vi "19_2.vi"() -> ()   [LabVIEW 2018]
uses:
  <userlib>/_OpenG.lib/array/array.llb/Remove Duplicates from 1D Array (String)__ogtk.vi
  <vilib>/regexp/Match Regular Expression.xnode
panel:
  out "size(s)":i32=311
  out "Array":i16[](array[numeric])=[190, 18, 8, 3, 0, 0, 0, 0, 0, 0, 37, 9, 0, 0, 0, 0, 0, 0, 0, 0, 23, 7, 0, 0, 0, 0, 0, 0, 0, 0, 10, 1, 0, 0, 0, 0, 0, 0, 0, 0, 5, 0, 0, 0, 0, 0, 0, 0, 0, 0, 0, 0, 0, 0, 0, 0, 0, 0, 0, 0, 0, 0, 0, 0, 0, 0, 0, 0, 0, 0, 0, 0, 0, 0, 0, 0, 0, 0, 0, 0, 0, 0, 0, 0, 0, 0, 0, 0, 0, 0, 0, 0, 0, 0, 0, 0, 0, 0, 0, 0]
  out "sum":i16
  out "String":string="((((a((a(b(aa|ba)|a(ab|aa))|b(b(bb|aa)|a(ba)))a|(((ab|ba)b)b|((aa|ba)b|((a|b)(a|b))a)a)b)|b((a(a(ba|a(a|b))|b((a|b)(a|b)))|b((ba)b|(bb|aa)a))a|((b(bb)|a(ab|ba))b|(b(bb|aa)|a(ba))a)b))a|(b(b(a(b(bb|aa)|a(ab|ba))|b(b(bb|aa)|a(ba)))|a(((bb)a|(bb|aa)b)a|((bb|aa)a|(aa|ba)b)b))|a(a(b(a(bb|aa)|b(aa|ba))|a((bb|ab)a|((a|b)b|ba)b))|b((a(aa|ba))a|((b(a|b)|aa)b|(ba)a)b)))b)a|(a(a(a((b(ba)|a(bb|aa))b|(b(bb|ab)|a(aa))a)|b(((bb|ab)b|(b(a|b)|aa)a)b|(b(bb|aa)|a(ab|ba))a))|b((a((b(a|b)|aa)b|(ba)a)|b((ba|bb)b|(ba|a(a|b))a))a|(b(b(ba)|a(bb|ab))|a((ba)b|(bb|aa)a))b))|b(a((((ba|bb)b|(ab|aa)a)a|((ba|a(a|b))(a|b))b)b|(((aa|ba)a|(ba|a(a|b))b)b|(a(aa|ba)|b(aa))a)a)|b((a(b((a|b)(a|b))|a(aa|ba))|b((ab|ba)b|(bb|ab)a))a|(a((ba|bb)a|(b(a|b)|aa)b)|b(((a|b)(a|b))b|(ba)a))b)))b)(((a((a(b(aa|ba)|a(ab|aa))|b(b(bb|aa)|a(ba)))a|(((ab|ba)b)b|((aa|ba)b|((a|b)(a|b))a)a)b)|b((a(a(ba|a(a|b))|b((a|b)(a|b)))|b((ba)b|(bb|aa)a))a|((b(bb)|a(ab|ba))b|(b(bb|aa)|a(ba))a)b))a|(b(b(a(b(bb|aa)|a(ab|ba))|b(b(bb|aa)|a(ba)))|a(((bb)a|(bb|aa)b)a|((bb|aa)a|(aa|ba)b)b))|a(a(b(a(bb|aa)|b(aa|ba))|a((bb|ab)a|((a|b)b|ba)b))|b((a(aa|ba))a|((b(a|b)|aa)b|(ba)a)b)))b)a|(a(a(a((b(ba)|a(bb|aa))b|(b(bb|ab)|a(aa))a)|b(((bb|ab)b|(b(a|b)|aa)a)b|(b(bb|aa)|a(ab|ba))a))|b((a((b(a|b)|aa)b|(ba)a)|b((ba|bb)b|(ba|a(a|b))a))a|(b(b(ba)|a(bb|ab))|a((ba)b|(bb|aa)a))b))|b(a((((ba|bb)b|(ab|aa)a)a|((ba|a(a|b))(a|b))b)b|(((aa|ba)a|(ba|a(a|b))b)b|(a(aa|ba)|b(aa))a)a)|b((a(b((a|b)(a|b))|a(aa|ba))|b((ab|ba)b|(bb|ab)a))a|(a((ba|bb)a|(b(a|b)|aa)b)|b(((a|b)(a|b))b|(ba)a))b)))b)(((a((a(b(aa|ba)|a(ab|aa))|b(b(bb|aa)|a(ba)))a|(((ab|ba)b)b|((aa|ba)b|((a|b)(a|b))a)a)b)|b((a(a(ba|a(a|b))|b((a|b)(a|b)))|b((ba)b|(bb|aa)a))a|((b(bb)|a(ab|ba))b|(b(bb|aa)|a(ba))a)b))a|(b(b(a(b(bb|aa)|a(ab|ba))|b(b(bb|aa)|a(ba)))|a(((bb)a|(bb|aa)b)a|((bb|aa)a|(aa|ba)b)b))|a(a(b(a(bb|aa)|b(aa|ba))|a((bb|ab)a|((a|b)b|ba)b))|b((a(aa|ba))a|((b(a|b)|aa)b|(ba)a)b)))b)a|(a(a(a((b(ba)|a(bb|aa))b|(b(bb|ab)|a(aa))a)|b(((bb|ab)b|(b(a|b)|aa)a)b|(b(bb|aa)|a(ab|ba))a))|b((a((b(a|b)|aa)b|(ba)a)|b((ba|bb)b|(ba|a(a|b))a))a|(b(b(ba)|a(bb|ab))|a((ba)b|(bb|aa)a))b))|b(a((((ba|bb)b|(ab|aa)a)a|((ba|a(a|b))(a|b))b)b|(((aa|ba)a|(ba|a(a|b))b)b|(a(aa|ba)|b(aa))a)a)|b((a(b((a|b)(a|b))|a(aa|ba))|b((ab|ba)b|(bb|ab)a))a|(a((ba|bb)a|(b(a|b)|aa)b)|b(((a|b)(a|b))b|(ba)a))b)))b)(((a((a(b(aa|ba)|a(ab|aa))|b(b(bb|aa)|a(ba)))a|(((ab|ba)b)b|((aa|ba)b|((a|b)(a|b))a)a)b)|b((a(a(ba|a(a|b))|b((a|b)(a|b)))|b((ba)b|(bb|aa)a))a|((b(bb)|a(ab|ba))b|(b(bb|aa)|a(ba))a)b))a|(b(b(a(b(bb|aa)|a(ab|ba))|b(b(bb|aa)|a(ba)))|a(((bb)a|(bb|aa)b)a|((bb|aa)a|(aa|ba)b)b))|a(a(b(a(bb|aa)|b(aa|ba))|a((bb|ab)a|((a|b)b|ba)b))|b((a(aa|ba))a|((b(a|b)|aa)b|(ba)a)b)))b)a|(a(a(a((b(ba)|a(bb|aa))b|(b(bb|ab)|a(aa))a)|b(((bb|ab)b|(b(a|b)|aa)a)b|(b(bb|aa)|a(ab|ba))a))|b((a((b(a|b)|aa)b|(ba)a)|b((ba|bb)b|(ba|a(a|b))a))a|(b(b(ba)|a(bb|ab))|a((ba)b|(bb|aa)a))b))|b(a((((ba|bb)b|(ab|aa)a)a|((ba|a(a|b))(a|b))b)b|(((aa|ba)a|(ba|a(a|b))b)b|(a(aa|ba)|b(aa))a)a)|b((a(b((a|b)(a|b))|a(aa|ba))|b((ab|ba)b|(bb|ab)a))a|(a((ba|bb)a|(b(a|b)|aa)b)|b(((a|b)(a|b))b|(ba)a))b)))b)(((a((a(b(aa|ba)|a(ab|aa))|b(b(bb|aa)|a(ba)))a|(((ab|ba)b)b|((aa|ba)b|((a|b)(a|b))a)a)b)|b((a(a(ba|a(a|b))|b((a|b)(a|b)))|b((ba)b|(bb|aa)a))a|((b(bb)|a(ab|ba))b|(b(bb|aa)|a(ba))a)b))a|(b(b(a(b(bb|aa)|a(ab|ba))|b(b(bb|aa)|a(ba)))|a(((bb)a|(bb|aa)b)a|((bb|aa)a|(aa|ba)b)b))|a(a(b(a(bb|aa)|b(aa|ba))|a((bb|ab)a|((a|b)b|ba)b))|b((a(aa|ba))a|((b(a|b)|aa)b|(ba)a)b)))b)a|(a(a(a((b(ba)|a(bb|aa))b|(b(bb|ab)|a(aa))a)|b(((bb|ab)b|(b(a|b)|aa)a)b|(b(bb|aa)|a(ab|ba))a))|b((a((b(a|b)|aa)b|(ba)a)|b((ba|bb)b|(ba|a(a|b))a))a|(b(b(ba)|a(bb|ab))|a((ba)b|(bb|aa)a))b))|b(a((((ba|bb)b|(ab|aa)a)a|((ba|a(a|b))(a|b))b)b|(((aa|ba)a|(ba|a(a|b))b)b|(a(aa|ba)|b(aa))a)a)|b((a(b((a|b)(a|b))|a(aa|ba))|b((ab|ba)b|(bb|ab)a))a|(a((ba|bb)a|(b(a|b)|aa)b)|b(((a|b)(a|b))b|(ba)a))b)))b)(((a((a(b(aa|ba)|a(ab|aa))|b(b(bb|aa)|a(ba)))a|(((ab|ba)b)b|((aa|ba)b|((a|b)(a|b))a)a)b)|b((a(a(ba|a(a|b))|b((a|b)(a|b)))|b((ba)b|(bb|aa)a))a|((b(bb)|a(ab|ba))b|(b(bb|aa)|a(ba))a)b))a|(b(b(a(b(bb|aa)|a(ab|ba))|b(b(bb|aa)|a(ba)))|a(((bb)a|(bb|aa)b)a|((bb|aa)a|(aa|ba)b)b))|a(a(b(a(bb|aa)|b(aa|ba))|a((bb|ab)a|((a|b)b|ba)b))|b((a(aa|ba))a|((b(a|b)|aa)b|(ba)a)b)))b)a|(a(a(a((b(ba)|a(bb|aa))b|(b(bb|ab)|a(aa))a)|b(((bb|ab)b|(b(a|b)|aa)a)b|(b(bb|aa)|a(ab|ba))a))|b((a((b(a|b)|aa)b|(ba)a)|b((ba|bb)b|(ba|a(a|b))a))a|(b(b(ba)|a(bb|ab))|a((ba)b|(bb|aa)a))b))|b(a((((ba|bb)b|(ab|aa)a)a|((ba|a(a|b))(a|b))b)b|(((aa|ba)a|(ba|a(a|b))b)b|(a(aa|ba)|b(aa))a)a)|b((a(b((a|b)(a|b))|a(aa|ba))|b((ab|ba)b|(bb|ab)a))a|(a((ba|bb)a|(b(a|b)|aa)b)|b(((a|b)(a|b))b|(ba)a))b)))b)(((a((a(b(aa|ba)|a(ab|aa))|b(b(bb|aa)|a(ba)))a|(((ab|ba)b)b|((aa|ba)b|((a|b)(a|b))a)a)b)|b((a(a(ba|a(a|b))|b((a|b)(a|b)))|b((ba)b|(bb|aa)a))a|((b(bb)|a(ab|ba))b|(b(bb|aa)|a(ba))a)b))a|(b(b(a(b(bb|aa)|a(ab|ba))|b(b(bb|aa)|a(ba)))|a(((bb)a|(bb|aa)b)a|((bb|aa)a|(aa|ba)b)b))|a(a(b(a(bb|aa)|b(aa|ba))|a((bb|ab)a|((a|b)b|ba)b))|b((a(aa|ba))a|((b(a|b)|aa)b|(ba)a)b)))b)a|(a(a(a((b(ba)|a(bb|aa))b|(b(bb|ab)|a(aa))a)|b(((bb|ab)b|(b(a|b)|aa)a)b|(b(bb|aa)|a(ab|ba))a))|b((a((b(a|b)|aa)b|(ba)a)|b((ba|bb)b|(ba|a(a|b))a))a|(b(b(ba)|a(bb|ab))|a((ba)b|(bb|aa)a))b))|b(a((((ba|bb)b|(ab|aa)a)a|((ba|a(a|b))(a|b))b)b|(((aa|ba)a|(ba|a(a|b))b)b|(a(aa|ba)|b(aa))a)a)|b((a(b((a|b)(a|b))|a(aa|ba))|b((ab|ba)b|(bb|ab)a))a|(a((ba|bb)a|(b(a|b)|aa)b)|b(((a|b)(a|b))b|(ba)a))b)))b)(((a((a(b(aa|ba)|a(ab|aa))|b(b(bb|aa)|a(ba)))a|(((ab|ba)b)b|((aa|ba)b|((a|b)(a|b))a)a)b)|b((a(a(ba|a(a|b))|b((a|b)(a|b)))|b((ba)b|(bb|aa)a))a|((b(bb)|a(ab|ba))b|(b(bb|aa)|a(ba))a)b))a|(b(b(a(b(bb|aa)|a(ab|ba))|b(b(bb|aa)|a(ba)))|a(((bb)a|(bb|aa)b)a|((bb|aa)a|(aa|ba)b)b))|a(a(b(a(bb|aa)|b(aa|ba))|a((bb|ab)a|((a|b)b|ba)b))|b((a(aa|ba))a|((b(a|b)|aa)b|(ba)a)b)))b)a|(a(a(a((b(ba)|a(bb|aa))b|(b(bb|ab)|a(aa))a)|b(((bb|ab)b|(b(a|b)|aa)a)b|(b(bb|aa)|a(ab|ba))a))|b((a((b(a|b)|aa)b|(ba)a)|b((ba|bb)b|(ba|a(a|b))a))a|(b(b(ba)|a(bb|ab))|a((ba)b|(bb|aa)a))b))|b(a((((ba|bb)b|(ab|aa)a)a|((ba|a(a|b))(a|b))b)b|(((aa|ba)a|(ba|a(a|b))b)b|(a(aa|ba)|b(aa))a)a)|b((a(b((a|b)(a|b))|a(aa|ba))|b((ab|ba)b|(bb|ab)a))a|(a((ba|bb)a|(b(a|b)|aa)b)|b(((a|b)(a|b))b|(ba)a))b)))b)(((a((a(b(aa|ba)|a(ab|aa))|b(b(bb|aa)|a(ba)))a|(((ab|ba)b)b|((aa|ba)b|((a|b)(a|b))a)a)b)|b((a(a(ba|a(a|b))|b((a|b)(a|b)))|b((ba)b|(bb|aa)a))a|((b(bb)|a(ab|ba))b|(b(bb|aa)|a(ba))a)b))a|(b(b(a(b(bb|aa)|a(ab|ba))|b(b(bb|aa)|a(ba)))|a(((bb)a|(bb|aa)b)a|((bb|aa)a|(aa|ba)b)b))|a(a(b(a(bb|aa)|b(aa|ba))|a((bb|ab)a|((a|b)b|ba)b))|b((a(aa|ba))a|((b(a|b)|aa)b|(ba)a)b)))b)a|(a(a(a((b(ba)|a(bb|aa))b|(b(bb|ab)|a(aa))a)|b(((bb|ab)b|(b(a|b)|aa)a)b|(b(bb|aa)|a(ab|ba))a))|b((a((b(a|b)|aa)b|(ba)a)|b((ba|bb)b|(ba|a(a|b))a))a|(b(b(ba)|a(bb|ab))|a((ba)b|(bb|aa)a))b))|b(a((((ba|bb)b|(ab|aa)a)a|((ba|a(a|b))(a|b))b)b|(((aa|ba)a|(ba|a(a|b))b)b|(a(aa|ba)|b(aa))a)a)|b((a(b((a|b)(a|b))|a(aa|ba))|b((ab|ba)b|(bb|ab)a))a|(a((ba|bb)a|(b(a|b)|aa)b)|b(((a|b)(a|b))b|(ba)a))b)))b)(((a((a(b(aa|ba)|a(ab|aa))|b(b(bb|aa)|a(ba)))a|(((ab|ba)b)b|((aa|ba)b|((a|b)(a|b))a)a)b)|b((a(a(ba|a(a|b))|b((a|b)(a|b)))|b((ba)b|(bb|aa)a))a|((b(bb)|a(ab|ba))b|(b(bb|aa)|a(ba))a)b))a|(b(b(a(b(bb|aa)|a(ab|ba))|b(b(bb|aa)|a(ba)))|a(((bb)a|(bb|aa)b)a|((bb|aa)a|(aa|ba)b)b))|a(a(b(a(bb|aa)|b(aa|ba))|a((bb|ab)a|((a|b)b|ba)b))|b((a(aa|ba))a|((b(a|b)|aa)b|(ba)a)b)))b)a|(a(a(a((b(ba)|a(bb|aa))b|(b(bb|ab)|a(aa))a)|b(((bb|ab)b|(b(a|b)|aa)a)b|(b(bb|aa)|a(ab|ba))a))|b((a((b(a|b)|aa)b|(ba)a)|b((ba|bb)b|(ba|a(a|b))a))a|(b(b(ba)|a(bb|ab))|a((ba)b|(bb|aa)a))b))|b(a((((ba|bb)b|(ab|aa)a)a|((ba|a(a|b))(a|b))b)b|(((aa|ba)a|(ba|a(a|b))b)b|(a(aa|ba)|b(aa))a)a)|b((a(b((a|b)(a|b))|a(aa|ba))|b((ab|ba)b|(bb|ab)a))a|(a((ba|bb)a|(b(a|b)|aa)b)|b(((a|b)(a|b))b|(ba)a))b)))b))((((a((a(b(aa|ba)|a(ab|aa))|b(b(bb|aa)|a(ba)))a|(((ab|ba)b)b|((aa|ba)b|((a|b)(a|b))a)a)b)|b((a(a(ba|a(a|b))|b((a|b)(a|b)))|b((ba)b|(bb|aa)a))a|((b(bb)|a(ab|ba))b|(b(bb|aa)|a(ba))a)b))a|(b(b(a(b(bb|aa)|a(ab|ba))|b(b(bb|aa)|a(ba)))|a(((bb)a|(bb|aa)b)a|((bb|aa)a|(aa|ba)b)b))|a(a(b(a(bb|aa)|b(aa|ba))|a((bb|ab)a|((a|b)b|ba)b))|b((a(aa|ba))a|((b(a|b)|aa)b|(ba)a)b)))b)a|(a(a(a((b(ba)|a(bb|aa))b|(b(bb|ab)|a(aa))a)|b(((bb|ab)b|(b(a|b)|aa)a)b|(b(bb|aa)|a(ab|ba))a))|b((a((b(a|b)|aa)b|(ba)a)|b((ba|bb)b|(ba|a(a|b))a))a|(b(b(ba)|a(bb|ab))|a((ba)b|(bb|aa)a))b))|b(a((((ba|bb)b|(ab|aa)a)a|((ba|a(a|b))(a|b))b)b|(((aa|ba)a|(ba|a(a|b))b)b|(a(aa|ba)|b(aa))a)a)|b((a(b((a|b)(a|b))|a(aa|ba))|b((ab|ba)b|(bb|ab)a))a|(a((ba|bb)a|(b(a|b)|aa)b)|b(((a|b)(a|b))b|(ba)a))b)))b)(((a((a(b(aa|ba)|a(ab|aa))|b(b(bb|aa)|a(ba)))a|(((ab|ba)b)b|((aa|ba)b|((a|b)(a|b))a)a)b)|b((a(a(ba|a(a|b))|b((a|b)(a|b)))|b((ba)b|(bb|aa)a))a|((b(bb)|a(ab|ba))b|(b(bb|aa)|a(ba))a)b))a|(b(b(a(b(bb|aa)|a(ab|ba))|b(b(bb|aa)|a(ba)))|a(((bb)a|(bb|aa)b)a|((bb|aa)a|(aa|ba)b)b))|a(a(b(a(bb|aa)|b(aa|ba))|a((bb|ab)a|((a|b)b|ba)b))|b((a(aa|ba))a|((b(a|b)|aa)b|(ba)a)b)))b)a|(a(a(a((b(ba)|a(bb|aa))b|(b(bb|ab)|a(aa))a)|b(((bb|ab)b|(b(a|b)|aa)a)b|(b(bb|aa)|a(ab|ba))a))|b((a((b(a|b)|aa)b|(ba)a)|b((ba|bb)b|(ba|a(a|b))a))a|(b(b(ba)|a(bb|ab))|a((ba)b|(bb|aa)a))b))|b(a((((ba|bb)b|(ab|aa)a)a|((ba|a(a|b))(a|b))b)b|(((aa|ba)a|(ba|a(a|b))b)b|(a(aa|ba)|b(aa))a)a)|b((a(b((a|b)(a|b))|a(aa|ba))|b((ab|ba)b|(bb|ab)a))a|(a((ba|bb)a|(b(a|b)|aa)b)|b(((a|b)(a|b))b|(ba)a))b)))b)(((a((a(b(aa|ba)|a(ab|aa))|b(b(bb|aa)|a(ba)))a|(((ab|ba)b)b|((aa|ba)b|((a|b)(a|b))a)a)b)|b((a(a(ba|a(a|b))|b((a|b)(a|b)))|b((ba)b|(bb|aa)a))a|((b(bb)|a(ab|ba))b|(b(bb|aa)|a(ba))a)b))a|(b(b(a(b(bb|aa)|a(ab|ba))|b(b(bb|aa)|a(ba)))|a(((bb)a|(bb|aa)b)a|((bb|aa)a|(aa|ba)b)b))|a(a(b(a(bb|aa)|b(aa|ba))|a((bb|ab)a|((a|b)b|ba)b))|b((a(aa|ba))a|((b(a|b)|aa)b|(ba)a)b)))b)a|(a(a(a((b(ba)|a(bb|aa))b|(b(bb|ab)|a(aa))a)|b(((bb|ab)b|(b(a|b)|aa)a)b|(b(bb|aa)|a(ab|ba))a))|b((a((b(a|b)|aa)b|(ba)a)|b((ba|bb)b|(ba|a(a|b))a))a|(b(b(ba)|a(bb|ab))|a((ba)b|(bb|aa)a))b))|b(a((((ba|bb)b|(ab|aa)a)a|((ba|a(a|b))(a|b))b)b|(((aa|ba)a|(ba|a(a|b))b)b|(a(aa|ba)|b(aa))a)a)|b((a(b((a|b)(a|b))|a(aa|ba))|b((ab|ba)b|(bb|ab)a))a|(a((ba|bb)a|(b(a|b)|aa)b)|b(((a|b)(a|b))b|(ba)a))b)))b)(((a((a(b(aa|ba)|a(ab|aa))|b(b(bb|aa)|a(ba)))a|(((ab|ba)b)b|((aa|ba)b|((a|b)(a|b))a)a)b)|b((a(a(ba|a(a|b))|b((a|b)(a|b)))|b((ba)b|(bb|aa)a))a|((b(bb)|a(ab|ba))b|(b(bb|aa)|a(ba))a)b))a|(b(b(a(b(bb|aa)|a(ab|ba))|b(b(bb|aa)|a(ba)))|a(((bb)a|(bb|aa)b)a|((bb|aa)a|(aa|ba)b)b))|a(a(b(a(bb|aa)|b(aa|ba))|a((bb|ab)a|((a|b)b|ba)b))|b((a(aa|ba))a|((b(a|b)|aa)b|(ba)a)b)))b)a|(a(a(a((b(ba)|a(bb|aa))b|(b(bb|ab)|a(aa))a)|b(((bb|ab)b|(b(a|b)|aa)a)b|(b(bb|aa)|a(ab|ba))a))|b((a((b(a|b)|aa)b|(ba)a)|b((ba|bb)b|(ba|a(a|b))a))a|(b(b(ba)|a(bb|ab))|a((ba)b|(bb|aa)a))b))|b(a((((ba|bb)b|(ab|aa)a)a|((ba|a(a|b))(a|b))b)b|(((aa|ba)a|(ba|a(a|b))b)b|(a(aa|ba)|b(aa))a)a)|b((a(b((a|b)(a|b))|a(aa|ba))|b((ab|ba)b|(bb|ab)a))a|(a((ba|bb)a|(b(a|b)|aa)b)|b(((a|b)(a|b))b|(ba)a))b)))b)(((a((a(b(aa|ba)|a(ab|aa))|b(b(bb|aa)|a(ba)))a|(((ab|ba)b)b|((aa|ba)b|((a|b)(a|b))a)a)b)|b((a(a(ba|a(a|b))|b((a|b)(a|b)))|b((ba)b|(bb|aa)a))a|((b(bb)|a(ab|ba))b|(b(bb|aa)|a(ba))a)b))a|(b(b(a(b(bb|aa)|a(ab|ba))|b(b(bb|aa)|a(ba)))|a(((bb)a|(bb|aa)b)a|((bb|aa)a|(aa|ba)b)b))|a(a(b(a(bb|aa)|b(aa|ba))|a((bb|ab)a|((a|b)b|ba)b))|b((a(aa|ba))a|((b(a|b)|aa)b|(ba)a)b)))b)a|(a(a(a((b(ba)|a(bb|aa))b|(b(bb|ab)|a(aa))a)|b(((bb|ab)b|(b(a|b)|aa)a)b|(b(bb|aa)|a(ab|ba))a))|b((a((b(a|b)|aa)b|(ba)a)|b((ba|bb)b|(ba|a(a|b))a))a|(b(b(ba)|a(bb|ab))|a((ba)b|(bb|aa)a))b))|b(a((((ba|bb)b|(ab|aa)a)a|((ba|a(a|b))(a|b))b)b|(((aa|ba)a|(ba|a(a|b))b)b|(a(aa|ba)|b(aa))a)a)|b((a(b((a|b)(a|b))|a(aa|ba))|b((ab|ba)b|(bb|ab)a))a|(a((ba|bb)a|(b(a|b)|aa)b)|b(((a|b)(a|b))b|(ba)a))b)))b)(((a((a(b(aa|ba)|a(ab|aa))|b(b(bb|aa)|a(ba)))a|(((ab|ba)b)b|((aa|ba)b|((a|b)(a|b))a)a)b)|b((a(a(ba|a(a|b))|b((a|b)(a|b)))|b((ba)b|(bb|aa)a))a|((b(bb)|a(ab|ba))b|(b(bb|aa)|a(ba))a)b))a|(b(b(a(b(bb|aa)|a(ab|ba))|b(b(bb|aa)|a(ba)))|a(((bb)a|(bb|aa)b)a|((bb|aa)a|(aa|ba)b)b))|a(a(b(a(bb|aa)|b(aa|ba))|a((bb|ab)a|((a|b)b|ba)b))|b((a(aa|ba))a|((b(a|b)|aa)b|(ba)a)b)))b)a|(a(a(a((b(ba)|a(bb|aa))b|(b(bb|ab)|a(aa))a)|b(((bb|ab)b|(b(a|b)|aa)a)b|(b(bb|aa)|a(ab|ba))a))|b((a((b(a|b)|aa)b|(ba)a)|b((ba|bb)b|(ba|a(a|b))a))a|(b(b(ba)|a(bb|ab))|a((ba)b|(bb|aa)a))b))|b(a((((ba|bb)b|(ab|aa)a)a|((ba|a(a|b))(a|b))b)b|(((aa|ba)a|(ba|a(a|b))b)b|(a(aa|ba)|b(aa))a)a)|b((a(b((a|b)(a|b))|a(aa|ba))|b((ab|ba)b|(bb|ab)a))a|(a((ba|bb)a|(b(a|b)|aa)b)|b(((a|b)(a|b))b|(ba)a))b)))b)(((a((a(b(aa|ba)|a(ab|aa))|b(b(bb|aa)|a(ba)))a|(((ab|ba)b)b|((aa|ba)b|((a|b)(a|b))a)a)b)|b((a(a(ba|a(a|b))|b((a|b)(a|b)))|b((ba)b|(bb|aa)a))a|((b(bb)|a(ab|ba))b|(b(bb|aa)|a(ba))a)b))a|(b(b(a(b(bb|aa)|a(ab|ba))|b(b(bb|aa)|a(ba)))|a(((bb)a|(bb|aa)b)a|((bb|aa)a|(aa|ba)b)b))|a(a(b(a(bb|aa)|b(aa|ba))|a((bb|ab)a|((a|b)b|ba)b))|b((a(aa|ba))a|((b(a|b)|aa)b|(ba)a)b)))b)a|(a(a(a((b(ba)|a(bb|aa))b|(b(bb|ab)|a(aa))a)|b(((bb|ab)b|(b(a|b)|aa)a)b|(b(bb|aa)|a(ab|ba))a))|b((a((b(a|b)|aa)b|(ba)a)|b((ba|bb)b|(ba|a(a|b))a))a|(b(b(ba)|a(bb|ab))|a((ba)b|(bb|aa)a))b))|b(a((((ba|bb)b|(ab|aa)a)a|((ba|a(a|b))(a|b))b)b|(((aa|ba)a|(ba|a(a|b))b)b|(a(aa|ba)|b(aa))a)a)|b((a(b((a|b)(a|b))|a(aa|ba))|b((ab|ba)b|(bb|ab)a))a|(a((ba|bb)a|(b(a|b)|aa)b)|b(((a|b)(a|b))b|(ba)a))b)))b)(((a((a(b(aa|ba)|a(ab|aa))|b(b(bb|aa)|a(ba)))a|(((ab|ba)b)b|((aa|ba)b|((a|b)(a|b))a)a)b)|b((a(a(ba|a(a|b))|b((a|b)(a|b)))|b((ba)b|(bb|aa)a))a|((b(bb)|a(ab|ba))b|(b(bb|aa)|a(ba))a)b))a|(b(b(a(b(bb|aa)|a(ab|ba))|b(b(bb|aa)|a(ba)))|a(((bb)a|(bb|aa)b)a|((bb|aa)a|(aa|ba)b)b))|a(a(b(a(bb|aa)|b(aa|ba))|a((bb|ab)a|((a|b)b|ba)b))|b((a(aa|ba))a|((b(a|b)|aa)b|(ba)a)b)))b)a|(a(a(a((b(ba)|a(bb|aa))b|(b(bb|ab)|a(aa))a)|b(((bb|ab)b|(b(a|b)|aa)a)b|(b(bb|aa)|a(ab|ba))a))|b((a((b(a|b)|aa)b|(ba)a)|b((ba|bb)b|(ba|a(a|b))a))a|(b(b(ba)|a(bb|ab))|a((ba)b|(bb|aa)a))b))|b(a((((ba|bb)b|(ab|aa)a)a|((ba|a(a|b))(a|b))b)b|(((aa|ba)a|(ba|a(a|b))b)b|(a(aa|ba)|b(aa))a)a)|b((a(b((a|b)(a|b))|a(aa|ba))|b((ab|ba)b|(bb|ab)a))a|(a((ba|bb)a|(b(a|b)|aa)b)|b(((a|b)(a|b))b|(ba)a))b)))b)(((a((a(b(aa|ba)|a(ab|aa))|b(b(bb|aa)|a(ba)))a|(((ab|ba)b)b|((aa|ba)b|((a|b)(a|b))a)a)b)|b((a(a(ba|a(a|b))|b((a|b)(a|b)))|b((ba)b|(bb|aa)a))a|((b(bb)|a(ab|ba))b|(b(bb|aa)|a(ba))a)b))a|(b(b(a(b(bb|aa)|a(ab|ba))|b(b(bb|aa)|a(ba)))|a(((bb)a|(bb|aa)b)a|((bb|aa)a|(aa|ba)b)b))|a(a(b(a(bb|aa)|b(aa|ba))|a((bb|ab)a|((a|b)b|ba)b))|b((a(aa|ba))a|((b(a|b)|aa)b|(ba)a)b)))b)a|(a(a(a((b(ba)|a(bb|aa))b|(b(bb|ab)|a(aa))a)|b(((bb|ab)b|(b(a|b)|aa)a)b|(b(bb|aa)|a(ab|ba))a))|b((a((b(a|b)|aa)b|(ba)a)|b((ba|bb)b|(ba|a(a|b))a))a|(b(b(ba)|a(bb|ab))|a((ba)b|(bb|aa)a))b))|b(a((((ba|bb)b|(ab|aa)a)a|((ba|a(a|b))(a|b))b)b|(((aa|ba)a|(ba|a(a|b))b)b|(a(aa|ba)|b(aa))a)a)|b((a(b((a|b)(a|b))|a(aa|ba))|b((ab|ba)b|(bb|ab)a))a|(a((ba|bb)a|(b(a|b)|aa)b)|b(((a|b)(a|b))b|(ba)a))b)))b)(((a((a(b(aa|ba)|a(ab|aa))|b(b(bb|aa)|a(ba)))a|(((ab|ba)b)b|((aa|ba)b|((a|b)(a|b))a)a)b)|b((a(a(ba|a(a|b))|b((a|b)(a|b)))|b((ba)b|(bb|aa)a))a|((b(bb)|a(ab|ba))b|(b(bb|aa)|a(ba))a)b))a|(b(b(a(b(bb|aa)|a(ab|ba))|b(b(bb|aa)|a(ba)))|a(((bb)a|(bb|aa)b)a|((bb|aa)a|(aa|ba)b)b))|a(a(b(a(bb|aa)|b(aa|ba))|a((bb|ab)a|((a|b)b|ba)b))|b((a(aa|ba))a|((b(a|b)|aa)b|(ba)a)b)))b)a|(a(a(a((b(ba)|a(bb|aa))b|(b(bb|ab)|a(aa))a)|b(((bb|ab)b|(b(a|b)|aa)a)b|(b(bb|aa)|a(ab|ba))a))|b((a((b(a|b)|aa)b|(ba)a)|b((ba|bb)b|(ba|a(a|b))a))a|(b(b(ba)|a(bb|ab))|a((ba)b|(bb|aa)a))b))|b(a((((ba|bb)b|(ab|aa)a)a|((ba|a(a|b))(a|b))b)b|(((aa|ba)a|(ba|a(a|b))b)b|(a(aa|ba)|b(aa))a)a)|b((a(b((a|b)(a|b))|a(aa|ba))|b((ab|ba)b|(bb|ab)a))a|(a((ba|bb)a|(b(a|b)|aa)b)|b(((a|b)(a|b))b|(ba)a))b)))b)(((((a(b(ba)|a(bb|aa))|b(b(aa|ba)|a(bb|ab)))a|(((ba|bb)b)b|(b(ba)|a((a|b)(a|b)))a)b)b|((((ba|a(a|b))(a|b))b|((ba|a(a|b))a|(ba)b)a)b|((b(bb)|a(ab|ba))a|(b(bb|ab)|a(aa))b)a)a)a|(a(a((((a|b)(a|b))a|(ab)b)b|((ab)a|(aa|ba)b)a)|b(a(b(bb|aa)|a((a|b)b|ba))|b((ba|bb)b|(ba|a(a|b))a)))|b(a(((bb)b|(bb)a)b|(b(aa|ba)|a(bb|ab))a)|b(((aa)b)b|((aa|ba)a|(b(a|b)|aa)b)a)))b)b|(((b(b(b(ab|aa)|a((a|b)b|ba))|a(a(ba|a(a|b))|b(ba|bb)))|a(a((ba|a(a|b))b|(bb)a)|b((b(a|b)|aa)b|(bb)a)))b|((b((b(a|b)|aa)b|(ba)a)|a(((a|b)b|ba)a|(ba|a(a|b))b))b|((b(ba)|a(bb|aa))b|(b(bb)|a(ba))a)a)a)a|(((b(a(ab|ba)|b((a|b)b|ba))|a((ba|a(a|b))a|((a|b)b|ba)b))a|(b(b(aa|ba)|a(bb|ab))|a((ab|ba)b))b)b|((a((ba|bb)b|((a|b)b|ba)a)|b(a(ab|ba)|b(bb|ab)))b|(b(((a|b)(a|b))a|(aa)b)|a((bb|aa)(a|b)))a)a)b)a)(((((a(b(ba)|a(bb|aa))|b(b(aa|ba)|a(bb|ab)))a|(((ba|bb)b)b|(b(ba)|a((a|b)(a|b)))a)b)b|((((ba|a(a|b))(a|b))b|((ba|a(a|b))a|(ba)b)a)b|((b(bb)|a(ab|ba))a|(b(bb|ab)|a(aa))b)a)a)a|(a(a((((a|b)(a|b))a|(ab)b)b|((ab)a|(aa|ba)b)a)|b(a(b(bb|aa)|a((a|b)b|ba))|b((ba|bb)b|(ba|a(a|b))a)))|b(a(((bb)b|(bb)a)b|(b(aa|ba)|a(bb|ab))a)|b(((aa)b)b|((aa|ba)a|(b(a|b)|aa)b)a)))b)b|(((b(b(b(ab|aa)|a((a|b)b|ba))|a(a(ba|a(a|b))|b(ba|bb)))|a(a((ba|a(a|b))b|(bb)a)|b((b(a|b)|aa)b|(bb)a)))b|((b((b(a|b)|aa)b|(ba)a)|a(((a|b)b|ba)a|(ba|a(a|b))b))b|((b(ba)|a(bb|aa))b|(b(bb)|a(ba))a)a)a)a|(((b(a(ab|ba)|b((a|b)b|ba))|a((ba|a(a|b))a|((a|b)b|ba)b))a|(b(b(aa|ba)|a(bb|ab))|a((ab|ba)b))b)b|((a((ba|bb)b|((a|b)b|ba)a)|b(a(ab|ba)|b(bb|ab)))b|(b(((a|b)(a|b))a|(aa)b)|a((bb|aa)(a|b)))a)a)b)a)(((((a(b(ba)|a(bb|aa))|b(b(aa|ba)|a(bb|ab)))a|(((ba|bb)b)b|(b(ba)|a((a|b)(a|b)))a)b)b|((((ba|a(a|b))(a|b))b|((ba|a(a|b))a|(ba)b)a)b|((b(bb)|a(ab|ba))a|(b(bb|ab)|a(aa))b)a)a)a|(a(a((((a|b)(a|b))a|(ab)b)b|((ab)a|(aa|ba)b)a)|b(a(b(bb|aa)|a((a|b)b|ba))|b((ba|bb)b|(ba|a(a|b))a)))|b(a(((bb)b|(bb)a)b|(b(aa|ba)|a(bb|ab))a)|b(((aa)b)b|((aa|ba)a|(b(a|b)|aa)b)a)))b)b|(((b(b(b(ab|aa)|a((a|b)b|ba))|a(a(ba|a(a|b))|b(ba|bb)))|a(a((ba|a(a|b))b|(bb)a)|b((b(a|b)|aa)b|(bb)a)))b|((b((b(a|b)|aa)b|(ba)a)|a(((a|b)b|ba)a|(ba|a(a|b))b))b|((b(ba)|a(bb|aa))b|(b(bb)|a(ba))a)a)a)a|(((b(a(ab|ba)|b((a|b)b|ba))|a((ba|a(a|b))a|((a|b)b|ba)b))a|(b(b(aa|ba)|a(bb|ab))|a((ab|ba)b))b)b|((a((ba|bb)b|((a|b)b|ba)a)|b(a(ab|ba)|b(bb|ab)))b|(b(((a|b)(a|b))a|(aa)b)|a((bb|aa)(a|b)))a)a)b)a)(((((a(b(ba)|a(bb|aa))|b(b(aa|ba)|a(bb|ab)))a|(((ba|bb)b)b|(b(ba)|a((a|b)(a|b)))a)b)b|((((ba|a(a|b))(a|b))b|((ba|a(a|b))a|(ba)b)a)b|((b(bb)|a(ab|ba))a|(b(bb|ab)|a(aa))b)a)a)a|(a(a((((a|b)(a|b))a|(ab)b)b|((ab)a|(aa|ba)b)a)|b(a(b(bb|aa)|a((a|b)b|ba))|b((ba|bb)b|(ba|a(a|b))a)))|b(a(((bb)b|(bb)a)b|(b(aa|ba)|a(bb|ab))a)|b(((aa)b)b|((aa|ba)a|(b(a|b)|aa)b)a)))b)b|(((b(b(b(ab|aa)|a((a|b)b|ba))|a(a(ba|a(a|b))|b(ba|bb)))|a(a((ba|a(a|b))b|(bb)a)|b((b(a|b)|aa)b|(bb)a)))b|((b((b(a|b)|aa)b|(ba)a)|a(((a|b)b|ba)a|(ba|a(a|b))b))b|((b(ba)|a(bb|aa))b|(b(bb)|a(ba))a)a)a)a|(((b(a(ab|ba)|b((a|b)b|ba))|a((ba|a(a|b))a|((a|b)b|ba)b))a|(b(b(aa|ba)|a(bb|ab))|a((ab|ba)b))b)b|((a((ba|bb)b|((a|b)b|ba)a)|b(a(ab|ba)|b(bb|ab)))b|(b(((a|b)(a|b))a|(aa)b)|a((bb|aa)(a|b)))a)a)b)a)(((((a(b(ba)|a(bb|aa))|b(b(aa|ba)|a(bb|ab)))a|(((ba|bb)b)b|(b(ba)|a((a|b)(a|b)))a)b)b|((((ba|a(a|b))(a|b))b|((ba|a(a|b))a|(ba)b)a)b|((b(bb)|a(ab|ba))a|(b(bb|ab)|a(aa))b)a)a)a|(a(a((((a|b)(a|b))a|(ab)b)b|((ab)a|(aa|ba)b)a)|b(a(b(bb|aa)|a((a|b)b|ba))|b((ba|bb)b|(ba|a(a|b))a)))|b(a(((bb)b|(bb)a)b|(b(aa|ba)|a(bb|ab))a)|b(((aa)b)b|((aa|ba)a|(b(a|b)|aa)b)a)))b)b|(((b(b(b(ab|aa)|a((a|b)b|ba))|a(a(ba|a(a|b))|b(ba|bb)))|a(a((ba|a(a|b))b|(bb)a)|b((b(a|b)|aa)b|(bb)a)))b|((b((b(a|b)|aa)b|(ba)a)|a(((a|b)b|ba)a|(ba|a(a|b))b))b|((b(ba)|a(bb|aa))b|(b(bb)|a(ba))a)a)a)a|(((b(a(ab|ba)|b((a|b)b|ba))|a((ba|a(a|b))a|((a|b)b|ba)b))a|(b(b(aa|ba)|a(bb|ab))|a((ab|ba)b))b)b|((a((ba|bb)b|((a|b)b|ba)a)|b(a(ab|ba)|b(bb|ab)))b|(b(((a|b)(a|b))a|(aa)b)|a((bb|aa)(a|b)))a)a)b)a)(((((a(b(ba)|a(bb|aa))|b(b(aa|ba)|a(bb|ab)))a|(((ba|bb)b)b|(b(ba)|a((a|b)(a|b)))a)b)b|((((ba|a(a|b))(a|b))b|((ba|a(a|b))a|(ba)b)a)b|((b(bb)|a(ab|ba))a|(b(bb|ab)|a(aa))b)a)a)a|(a(a((((a|b)(a|b))a|(ab)b)b|((ab)a|(aa|ba)b)a)|b(a(b(bb|aa)|a((a|b)b|ba))|b((ba|bb)b|(ba|a(a|b))a)))|b(a(((bb)b|(bb)a)b|(b(aa|ba)|a(bb|ab))a)|b(((aa)b)b|((aa|ba)a|(b(a|b)|aa)b)a)))b)b|(((b(b(b(ab|aa)|a((a|b)b|ba))|a(a(ba|a(a|b))|b(ba|bb)))|a(a((ba|a(a|b))b|(bb)a)|b((b(a|b)|aa)b|(bb)a)))b|((b((b(a|b)|aa)b|(ba)a)|a(((a|b)b|ba)a|(ba|a(a|b))b))b|((b(ba)|a(bb|aa))b|(b(bb)|a(ba))a)a)a)a|(((b(a(ab|ba)|b((a|b)b|ba))|a((ba|a(a|b))a|((a|b)b|ba)b))a|(b(b(aa|ba)|a(bb|ab))|a((ab|ba)b))b)b|((a((ba|bb)b|((a|b)b|ba)a)|b(a(ab|ba)|b(bb|ab)))b|(b(((a|b)(a|b))a|(aa)b)|a((bb|aa)(a|b)))a)a)b)a)(((((a(b(ba)|a(bb|aa))|b(b(aa|ba)|a(bb|ab)))a|(((ba|bb)b)b|(b(ba)|a((a|b)(a|b)))a)b)b|((((ba|a(a|b))(a|b))b|((ba|a(a|b))a|(ba)b)a)b|((b(bb)|a(ab|ba))a|(b(bb|ab)|a(aa))b)a)a)a|(a(a((((a|b)(a|b))a|(ab)b)b|((ab)a|(aa|ba)b)a)|b(a(b(bb|aa)|a((a|b)b|ba))|b((ba|bb)b|(ba|a(a|b))a)))|b(a(((bb)b|(bb)a)b|(b(aa|ba)|a(bb|ab))a)|b(((aa)b)b|((aa|ba)a|(b(a|b)|aa)b)a)))b)b|(((b(b(b(ab|aa)|a((a|b)b|ba))|a(a(ba|a(a|b))|b(ba|bb)))|a(a((ba|a(a|b))b|(bb)a)|b((b(a|b)|aa)b|(bb)a)))b|((b((b(a|b)|aa)b|(ba)a)|a(((a|b)b|ba)a|(ba|a(a|b))b))b|((b(ba)|a(bb|aa))b|(b(bb)|a(ba))a)a)a)a|(((b(a(ab|ba)|b((a|b)b|ba))|a((ba|a(a|b))a|((a|b)b|ba)b))a|(b(b(aa|ba)|a(bb|ab))|a((ab|ba)b))b)b|((a((ba|bb)b|((a|b)b|ba)a)|b(a(ab|ba)|b(bb|ab)))b|(b(((a|b)(a|b))a|(aa)b)|a((bb|aa)(a|b)))a)a)b)a)(((((a(b(ba)|a(bb|aa))|b(b(aa|ba)|a(bb|ab)))a|(((ba|bb)b)b|(b(ba)|a((a|b)(a|b)))a)b)b|((((ba|a(a|b))(a|b))b|((ba|a(a|b))a|(ba)b)a)b|((b(bb)|a(ab|ba))a|(b(bb|ab)|a(aa))b)a)a)a|(a(a((((a|b)(a|b))a|(ab)b)b|((ab)a|(aa|ba)b)a)|b(a(b(bb|aa)|a((a|b)b|ba))|b((ba|bb)b|(ba|a(a|b))a)))|b(a(((bb)b|(bb)a)b|(b(aa|ba)|a(bb|ab))a)|b(((aa)b)b|((aa|ba)a|(b(a|b)|aa)b)a)))b)b|(((b(b(b(ab|aa)|a((a|b)b|ba))|a(a(ba|a(a|b))|b(ba|bb)))|a(a((ba|a(a|b))b|(bb)a)|b((b(a|b)|aa)b|(bb)a)))b|((b((b(a|b)|aa)b|(ba)a)|a(((a|b)b|ba)a|(ba|a(a|b))b))b|((b(ba)|a(bb|aa))b|(b(bb)|a(ba))a)a)a)a|(((b(a(ab|ba)|b((a|b)b|ba))|a((ba|a(a|b))a|((a|b)b|ba)b))a|(b(b(aa|ba)|a(bb|ab))|a((ab|ba)b))b)b|((a((ba|bb)b|((a|b)b|ba)a)|b(a(ab|ba)|b(bb|ab)))b|(b(((a|b)(a|b))a|(aa)b)|a((bb|aa)(a|b)))a)a)b)a)(((((a(b(ba)|a(bb|aa))|b(b(aa|ba)|a(bb|ab)))a|(((ba|bb)b)b|(b(ba)|a((a|b)(a|b)))a)b)b|((((ba|a(a|b))(a|b))b|((ba|a(a|b))a|(ba)b)a)b|((b(bb)|a(ab|ba))a|(b(bb|ab)|a(aa))b)a)a)a|(a(a((((a|b)(a|b))a|(ab)b)b|((ab)a|(aa|ba)b)a)|b(a(b(bb|aa)|a((a|b)b|ba))|b((ba|bb)b|(ba|a(a|b))a)))|b(a(((bb)b|(bb)a)b|(b(aa|ba)|a(bb|ab))a)|b(((aa)b)b|((aa|ba)a|(b(a|b)|aa)b)a)))b)b|(((b(b(b(ab|aa)|a((a|b)b|ba))|a(a(ba|a(a|b))|b(ba|bb)))|a(a((ba|a(a|b))b|(bb)a)|b((b(a|b)|aa)b|(bb)a)))b|((b((b(a|b)|aa)b|(ba)a)|a(((a|b)b|ba)a|(ba|a(a|b))b))b|((b(ba)|a(bb|aa))b|(b(bb)|a(ba))a)a)a)a|(((b(a(ab|ba)|b((a|b)b|ba))|a((ba|a(a|b))a|((a|b)b|ba)b))a|(b(b(aa|ba)|a(bb|ab))|a((ab|ba)b))b)b|((a((ba|bb)b|((a|b)b|ba)a)|b(a(ab|ba)|b(bb|ab)))b|(b(((a|b)(a|b))a|(aa)b)|a((bb|aa)(a|b)))a)a)b)a)(((((a(b(ba)|a(bb|aa))|b(b(aa|ba)|a(bb|ab)))a|(((ba|bb)b)b|(b(ba)|a((a|b)(a|b)))a)b)b|((((ba|a(a|b))(a|b))b|((ba|a(a|b))a|(ba)b)a)b|((b(bb)|a(ab|ba))a|(b(bb|ab)|a(aa))b)a)a)a|(a(a((((a|b)(a|b))a|(ab)b)b|((ab)a|(aa|ba)b)a)|b(a(b(bb|aa)|a((a|b)b|ba))|b((ba|bb)b|(ba|a(a|b))a)))|b(a(((bb)b|(bb)a)b|(b(aa|ba)|a(bb|ab))a)|b(((aa)b)b|((aa|ba)a|(b(a|b)|aa)b)a)))b)b|(((b(b(b(ab|aa)|a((a|b)b|ba))|a(a(ba|a(a|b))|b(ba|bb)))|a(a((ba|a(a|b))b|(bb)a)|b((b(a|b)|aa)b|(bb)a)))b|((b((b(a|b)|aa)b|(ba)a)|a(((a|b)b|ba)a|(ba|a(a|b))b))b|((b(ba)|a(bb|aa))b|(b(bb)|a(ba))a)a)a)a|(((b(a(ab|ba)|b((a|b)b|ba))|a((ba|a(a|b))a|((a|b)b|ba)b))a|(b(b(aa|ba)|a(bb|ab))|a((ab|ba)b))b)b|((a((ba|bb)b|((a|b)b|ba)a)|b(a(ab|ba)|b(bb|ab)))b|(b(((a|b)(a|b))a|(aa)b)|a((bb|aa)(a|b)))a)a)b)a))"
  out "element":string="8 11"
  out "Rules":string[](array[string])=["62: 110 112 | 92 68", "85: 38 92 | 102 110", "63: 92 6 | 110 23", "82: 110 | 92", "99: 110 122 | 92 54", "33: 110 61 | 92 103", "24: 110 92 | 110 110", "76: 3 92", "109: 26 92 | 81 110", "94: 92 78 | 110 28", "17: 110 115", "61: 92 110 | 110 82", "25: 9 110 | 61 92", "114: 47 110 | 63 92", "21: 30 82", "103: 82 82", "69: 5 110 | 43 92", "73: 110 116 | 92 69", "52: 92 81 | 110 103", "22: 119 92 | 50 110", "108: 37 92 | 35 110", "2: 71 92 | 20 110", "119: 103 110 | 88 92", "102: 101 92 | 49 110", "92: b", "91: 92 54 | 110 3", "64: 92 115 | 110 24", "68: 92 30 | 110 81", "89: 115 110 | 26 92", "80: 61 110 | 81 92", "19: 110 73 | 92 1", "16: 115 92 | 103 110", "15: 123 110 | 58 92", "115: 110 110 | 92 110", "70: 92 30 | 110 9", "40: 110 96 | 92 99", "50: 88 110 | 115 92", "18: 26 92 | 48 110", "81: 92 110", "107: 110 30 | 92 115", "38: 84 110 | 12 92", "44: 40 92 | 66 110", "27: 125 92 | 2 110", "41: 92 128 | 110 118", "56: 81 92 | 30 110", "88: 110 92", "13: 75 92", "55: 75 110 | 26 92", "12: 13 92 | 52 110", "28: 122 92", "121: 75 92 | 24 110", "113: 92 81 | 110 54", "98: 103 110 | 3 92", "6: 92 62 | 110 126", "96: 75 92 | 9 110", "9: 82 92 | 92 110", "0: 8 11", "32: 104 92 | 91 110", "116: 110 32 | 92 67", "104: 92 81 | 110 30", "5: 110 109 | 92 105", "117: 110 22 | 92 59", "128: 92 24 | 110 9", "66: 92 98 | 110 21", "46: 76 92 | 89 110", "36: 92 90 | 110 127", "20: 110 115 | 92 3", "4: 48 110 | 30 92", "26: 92 82 | 110 110", "39: 30 110 | 115 92", "127: 61 110 | 9 92", "84: 110 104 | 92 78", "100: 97 92 | 68 110", "106: 110 7 | 92 18", "123: 110 64 | 92 68", "111: 110 74 | 92 46", "42: 114 110 | 19 92", "58: 28 92 | 16 110", "47: 110 15 | 92 124", "54: 92 92 | 110 92", "51: 110 117 | 92 111", "130: 92 41 | 110 106", "30: 92 92 | 110 110", "72: 17 110 | 109 92", "129: 130 92 | 108 110", "14: 85 110 | 51 92", "53: 87 92 | 44 110", "112: 92 30 | 110 122", "45: 61 82", "105: 75 92 | 61 110", "90: 110 122 | 92 9", "122: 110 92 | 92 110", "83: 110 33 | 92 56", "118: 110 61 | 92 75", "74: 120 92 | 78 110", "29: 110 65 | 92 60", "31: 14 92 | 10 110", "110: a", "87: 36 110 | 94 92", "57: 92 48 | 110 81", "78: 92 115 | 110 54", "97: 92 48 | 110 122", "1: 110 27 | 92 34", "95: 92 107 | 110 86", "79: 110 55 | 92 77", "37: 92 109 | 110 25", "126: 4 110 | 39 92", "101: 45 92 | 80 110", "59: 110 70 | 92 105", "7: 61 92 | 48 110", "48: 92 92", "35: 104 92 | 57 110", "120: 48 92 | 48 110", "34: 29 110 | 79 92", "93: 54 92 | 26 110", "71: 115 110 | 61 92", "125: 121 110 | 45 92", "60: 122 92 | 54 110", "86: 54 110 | 9 92", "49: 97 110 | 91 92", "3: 110 110", "23: 110 95 | 92 72", "65: 92 103 | 110 115", "10: 129 110 | 53 92", "8: 42", "11: 42 31", "77: 103 92 | 81 110", "67: 93 92 | 112 110", "75: 92 110 | 92 92", "124: 83 110 | 100 92", "43: 92 113 | 110 56"]
  out "Messages":string[](array[string])=["abbabbbbaaabbbbabbbababaaabaabaabbaabbba", "babaaaabbaaabbbbbbbbbaba", "bbbbaaaabaaabbabaababbbabaaaaaababaabaaaaabbabbb", "baabbbbbbbaababaababbbabbababbbbaaaabbbbbabaabbabaaababb", "aabbaabbbbbaabbbbaaabaab", "bbaaabbaaaabababbbbaabaa", "abbbbbababbaabaabaaaabbbaaaabaab", "abaabbbbabaaabaabbbbaabbabaabaaabbaaabbbabbaabbbaabbbabb", "baabbbbbaabbaaabbabbabaa", "babbabbbabaabaaaaabbababaaaabaaaabbababbabababbaaababaaa", "aaababaabababbbbabaaaaab", "bbabaabaabbaabaabbbbbbab", "bbbbaaaabaaabbabbbbbbaababaabbaabaabbaab", "aaabbabbbabababbaabbabba", "abbbbbbabbababbbbabbabbabbabaabbaaabbaab", "bbbbabaaabbaabbabaaabbbababababbabaabbaabbabbbaa", "aabaaaaabaabaaabaaabbaababbbaaababbbbbbabbbbabababbbabbaabaaabaa", "baaaababbaaaaaabaabbbabbaaabaaab", "abbabbbaaabaaabbaaaaabbb", "ababaaaababaaaaaaababbaa", "babbabbabbababababbaaabb", "bbabbaabaaabbabbababaaababababaaaaababaabbaababb", "bbababbbbbabaaabaaabaaaa", "abbaaabaaaabaabbbbbaaaba", "aaaabababbbbabaabaabaaabbabbabbabaaababaaabaabbaabaaabbabbaaaabababbbaab", "aabaababaaaaaabbaabaaabbbabbbaaabaabaaaaabbaaaba", "bababaaaabbaabbbaaaabbab", "abababaabbbbbaababbaaaabbabaabbbabbbbaaaabaaabbbabbbbaba", "ababababababbbaaababbbba", "ababbabbabaabbbaabaaaabbaaaaaaaaaaabaaaabbbababb", "aaabbabbbaaabaaaabaabaaa", "abbbbabbabbbbaaabbbbabbbbabaaaababbbabaababbaabbabaaabba", "bbbababaaaaabaaabaabaaabbaababba", "aaaabbbbbbabababbbaaabab", "aabaababbbbbaabaabaaabaaabababbbbababbabbbbabbaa", "babbabbaabababaaabbbabaa", "baaaaaaabbabababbbaabaaa", "aaababaaaaabaaaaabaaabbaabaaaaab", "abaaabaabaaabaabaaabaaaabbaabaaabbbbbbab", "aaabbbabaababbbbbaabaaba", "bababbbaabababaabababaab", "bababbbaaaabaaaabbbaaabbabbaaabb", "ababaaabbababaaabbabbbbabaabaabaabaababb", "bbabbaabbabaabbbabbabbbaaabbaabaaaaaaaababbbbaaaabbaabab", "aaababababaaaabbaaaaabba", "babaababbbbabababaabaaaaababbabaabaaabba", "aaaabaaaabababaaaaabbaaa", "aabaaaaababbbaaaabbbabababbabbaa", "bbbbaababaabbbabbbbabbaa", "baaaaaabaabaaaaaabbaabbaabbabbbbbbbabbabbbbbabbbabaabbab", "ababababbaaaaaabaabaabbb", "abbbababababbbaababbaabb", "aabbaaabaabbaabbaaaaaabbbbaaabbaabbbaaaa", "bbabbbbaaababaababbbbbbaabbbbbabbabbabbb", "babbbabaabaabbbabaabbaab", "bbabbbabababbbabaababbbaaabaaaababbbbaba", "babbaaaabbbabbbbabbaaaba", "bbbbababbbababbbbbabbbabbbaabbbbaaabbaaa", "ababbbaababbbabaaaaaaabaabaaaaaabbabaabbaaaaaabababaaabaaaaaababbbbabbbbaababbaabbbbaaab", "aabbbabbaabbaabbbaaabababaaabaabbbabbaba", "bbbabaabbbabbaabbaabaaaababbababababbbba", "abaabbbabaaaaabbabaaabbb", "bababbabaabaabaaaabbbbaabbababba", "aabbaaabaabbbabbaababaaa", "baababbbbbabaabaaaaabbab", "bbbbabbaabbbbbbbabbbaaaaaaabaabababaaaaaabababbbbaababab", "baaaabbabbaaaaaababaaaaaabaabbbbababbbbb", "baababbbabbbbaaabbaabaaa", "bbbabbabbbbbabbbbaaaaaaaaaabbabaabaababb", "bbbbbbaabaabbbaaabbbaaba", "bbbababaaabbbbbbbbbbababaabaabaababbbbba", "abbaabbaabbaaaababaaaaababaabaaaaabbbaabaabaaaabaabbabbbbabaabba", "baaaabbbaaabbaabaabbbabababbaaab", "abaaabaaabababaababbbbbb", "bbbbaaaabbabaabaabaaabaabaabbaaa", "bbaaabbbbaaaaaaabaabbbbbbbbaabbbaaaaabbb", "abbaabbabaaabbabaaabbbbabbababba", "baabaaaaaabbabaaaabaabbbbaabbaab", "babbbababaaababaabaabbaa", "aabbbbaaababbbaaabaaaaab", "bbaaabbbaabaaabaabbbabba", "babbbaaabababaaababbbaab", "aaaaaaaaabbbababaaabbaab", "bbaabaabbabbbaaababbbaaabbbbbaabbbababba", "ababababbaaabbabbababbbbbbbbabba", "abbaabbababbbabaabbabbbabbaaaaababbbabababaabbaa", "aabbbabaaaabbbbbababbbbbbabbaaabbabaababaabbabab", "babbbaaababaabbbbbbabbaa", "ababaabaaabbaaababaabbbb", "aabaabaaaabbbbaaaabbabaa", "baaaabbbbbbababbaabaababaabbabaaababbbbabaaabbbbbbbaaabbabbbbbbaaaaaaabaaaaaabbbbbbaaaba", "baaabbabbabbbabaaaabaaba", "baaaabbbbbbbbaababbbbbbb", "baaaabbaaabbbbbbaababaaa", "aabaababbaaaababaabbabba", "aabbbbaaaabbaaaabaababba", "bbaaabaaaaaabbbabbabaabababbabbaaababbababaabbab", "abbabbbaaabaaabbabbabbaa", "aaaaabbbbbbbbbbbabaababbababbbbabbbabbbaabaababb", "bbbbababbbabaabababbbabaaabaabababaaaabbabaabbabbbaabbab", "babbbabbbababbbbabbaabbbabaaaabbbbabbaabaabbabaaabbbbaab", "baabaabbaaababbaaababbbbbbaaabbbabaaaaabbbbbaaabbbbaaaaa", "abaaababaaaabababbaabbab", "abababaaaaaabaaababbabba", "abbbaaabbaabbbbbbaaababb", "baabbbbbbbbbabbbbbaabbba", "abaaabaaabbbbbabbbbabbba", "babbbabbaabaabaaabaaaaaa", "aaabbabbabaaababbbbabbabbabaaaabaabbababbbbbabba", "aabaaaaaababaaaabababaaaabbbbbbababbaabaabbbaaaa", "abaaaabbbbbabaaaaabbbbababaabaaa", "aaabbbabaaaabaaaabbabbab", "bbbbaabbbabbbabbbaaabbbabaabaabbbabbabbbabaaabbaabbababb", "babaabbbbbbbababbbaabaababbaaabb", "abbbbabbbbbbbbbababbaabb", "abaaaabbaabbbbaabaabbbbbbabbabbababbbbbbabbabbaabababaab", "aaabbabbaaaabbbaabbbabaa", "babbbabaabababaaababbaba", "abbaabbababaaaaaaababaaa", "aabbbabbabababbbabbbbbaa", "aababbbbbaaaaabbbaabbaab", "aabbaabaaabaabaaaabbbaab", "abaabbbabababaaaaabababb", "abbbbbbaabaaabaababbabbb", "baabaaaaaaabbabaaabbaabbaabbaaab", "baababbaababbaabbbbabbaa", "ababababbabaaaabbaaabaab", "abbabbbbabbbababaabababb", "bbabbabbbbabaaabaabbbbba", "aaaaaabbbaaaaabbabbababb", "baaabaaababbbabaaababbbbbbaabbab", "bbbbbbbababaababaababbaa", "baaaaaaaabaabbbaababbabbbaaaaaabbaabaaaaababbbbaaabaabaa", "aaabbbabbaaaabbbbabbbabababaaabababaabba", "bbbabbabababbabbbabaaabb", "bbaaabaaaaaaaaaababaaabb", "aabaabbaaabbbaabbaaabaaaababbaab", "abbbbaaabbabbbbbbbbbbbaabbabbabbbabbbbab", "aaababaabaababaabbbaabab", "baabaabbbbabbbabababbaaa", "abbbaaabaabaababbbbbababababbaabbabaaaaaabbbbbaa", "aabbbbbbbbbabbbbabaabaab", "bababaaabbbabbbbababbaba", "bbabaabbbababaaabaaaaabb", "bbbbbbaababaababababbbbb", "bababbbbabbbbbabbaabaaba", "aabaababbbbbbbbabaabbbabbbabbbabbbabbaabaabaaabbababbaba", "ababbbabbaaabbabababbbbbababaabaaabaabaabbbaaaaaaaaabbaabbbababbaaabbabbbbaabbaa", "bbabbbabaaabbabaabaabaaa", "bbabbaabbbaaaaabababbbbb", "bbbbbbaaababbabbaababbaa", "bbbbbbaabbabababaaaabaab", "abbaaabbabbababbabababbaaabbbbababbaabbbabbbbbab", "bbbbababbabbbabbbbaabaaa", "bbaabaabbababbaaaabbaaaabaaaaaba", "abbaabaaababbabbabbbabaaaaaabaab", "baaaababbbabbabbbbbbaabbabbaaaaabaabbbaaaaabbaaaabaaaaab", "bbbbbbbabaabaaabbbabbbbaaabbbbababbaaabb", "bbaaabaaabbaaaaaaaabbaaa", "babaabbbabbabbbbbaaabbbbababaabb", "bbbbabbbbababbbabbabbbaa", "baaaaaababbaaaabbbbaabba", "abbbaaabbbbbababaabbbbbb", "aabbaaaaaababaabbabaabbbbabbaabaaaaaaaaaaababbab", "aaabbabbbbbabababbbbbbab", "babaabaabbbabaaaaaabbababaababba", "abaabbbaabbbbbababaaaaab", "aaabbabbaabababbaabbbbba", "aabaaabaaaaabbbaabbbaabaababbbbbbbbbaabbbbbbaabbbaabbaaa", "abbaabbbbaaaabbbabbbaabb", "bbaaabbaaaababaabbbabaababaaaabaaabbbaabbbaababbbaababba", "babaababbabaaaaaaaaaabaabbbbbaababbabbaa", "bbaaabbabbabbbabaaaaabbb", "aaaabababbababbbaabbbbababbaaaaabaaaaaba", "bbabaabbbbbbbbbaabaaaaab", "bbabaaababaaababbaaaabaa", "aabbaaabaabbbabaabbbabaa", "bababaaabbbbbbbabababaaaabaaaaab", "abaaaabbaaaaababaaaaaaba", "baaaabbaaaababababaabaabbaaaaabbbaababba", "bbababbbbbaaaaabaabababb", "bbbabbbbbbbbaababbbbaabaabbbbbaa", "bbbabbbbabaabaaaababbbbaababaabb", "bbbbababbabbbabbbabbabaa", "baaabababaabbbaabbabaabababbabbaabbaabab", "aaababbabaaaaaaabbbaaaba", "baaaaaabaabaaabaaabaabba", "babbaabababababbaaabbaaa", "bbbababaaaaaaaabbbbaaaab", "bababbaabbbabaabbaaaaaba", "abababbbbbbbabababbabbaa", "aaabbbabbaaabbabaabababa", "aaaabbbababaabbbabbaaaaaabaababbbabbabab", "bbaaaaababaaabaababaaaabbabaabbbaaaabbaa", "abbabaabaabbaaabbababbbabaaabaab", "abbbababaaabbabbaaabbaab", "abbabbbbabaaababaaabbbaa", "aababaababbaabbbaababbaa", "babaabaaaaabaaabbbbbaaab", "aababbbbbaababbbbaabbabb", "bbbbaaaaabaaaaabbbbaabaabbababbabaaabbaabbbaabab", "ababababbaaaabbbbbbaabbbabbbbbaa", "bbabbbbbbbababbbbabbabab", "bbbbbbbbbbabbaabbabbbaaaaabbbabaaabbbbba", "bbabbbabaabbaaabbbbabbba", "aabaabbbbbaababbaabababa", "bbaabaabbbbbababbbbbbaaa", "bababbaaaaaaaabbabbbbaaabbbabaababbbbababbabbbaaabbbaabb", "aabbbbbbbbbbabaabbbbbaaa", "ababbbaabbbaabbbbaaaaaabababaaababbbababbbabababbbaabbbb", "aabbbbbbbaabbbabbbabbaaa", "bababbababaaaabbabaabbab", "aababbbbababababaaabbaaa", "bbbbababbbabbbabbaababaa", "abbbbaaabbaaabbbbaaaaabbaaaaabba", "abbaabbabbaabaabbabbaabb", "baaaabbbaaabbbbabaaabaab", "baaabaaabbaababaaaabbaab", "baabbbabbbbbbaabbabaabbbbaababab", "bbabababaaabbbababaababa", "aabaabaabbabbbbababbaaababbbabbbaabbabaabbbbabbabbbbbbbb", "abaaaababbbbababaabababb", "abbabbbbaaaabbbbabbabbbbababaabb", "aababaabaaaaabaababaaaba", "abbbbaaabbaaaaabaaabbaaa", "aabaaabaaabbaaaaaaaabaab", "bbaaabbbbbbababaaabababa", "bbbabbabbaaaababbabaabbbaabbbbbbabbaaaaabbababba", "bbbbababbaaaaabbabbbbbabbaabbabb", "bbabaabbbbbbaabbbaabbbabaabaaaaabaabbaaa", "abbaaaabbbbbabbbabaabaaa", "aaabbbbaaaababbabaaaaaba", "bababbaabaaaabbaaaabbaaa", "ababababaaaabaaaababbaab", "aabaaababbabaabaabaabbbb", "abbaabbbbbbbabbbbbbbbaabbbababbbaaabbaaabbababaa", "abbabbbbaaaabaaababbbabaabbbabaaaabbabaa", "aababbbbbaabaabbbbbabaabaababbbbbbbbaaabbbabbaaa", "babaaaabbbabbaabbaababba", "bbabbbabbbbbabaabaaaabaa", "aaaaaabbaabbbababaaabaab", "abaaaababbbbbbaaabaabaab", "abaabbbabaaaaabaaaaabbaaaaaababbabbbaabb", "bbbbaaaaabbaabbabbbbabbbbbabaabaaaabaaab", "bbabaaabaababbbabbababbbababbaaa", "bbbbbbbbbbabaaabbaabbabb", "bbbabbbbabbaabbbbaababbbabbababb", "bbaaabbabaabbbaabaababab", "bbabaabaabbbababbaaabbabbbbbaaab", "abbbbaaaababababbabaabbbabbbbbbb", "babaaaaaaabaaabababaababbabbaabbbbaabaaa", "baaaabbabbaababaabbababb", "aaaaaaabbaaaabbbbbbaaaaa", "aabaaaaabbbabaabbaababaa", "abbabaabbbabbbbbbaabaaaaaaaabbaaaaabbaab", "baaaabababbbbaaabaababaa", "babaaaaabaaabbbbaaabaaaa", "aaabbababaaaaaaaabbbabaa", "bbabaaabbaaaababaaabaaaa", "bbaaabbbbabbbbbaaabbbbbaaabbbbbabbabaabababbbbbaabbabbaabbbabbbaaaaaaaababbbbababaabaabb", "aabaaaaaaabababababbabaaaaabbaaa", "bbbabaaabbaaaaaabbbaaaab", "abaaaaaabbabaaaabbbaabbabbababaa", "bbaaabbaaabbbabaababbbbb", "bbabaaabbababbbababaaaabbabaaaba", "abbabbbabaaabbbaaabaaaab", "baaabbbbbabbbaaabbbaaabb", "bbaaabbaababbbababaaabba", "aaaaabaaaabbbbabaabbbbaaaababbbbbabaabbbbbabbbaa", "bbaaaaaaabababbbbabbbbaa", "ababbabbaabaaaaaaaababbb", "babbabbabaabaaabbabaababbbbaabbbbbababababaababb", "abbaaaaabababbbbaaaabababbaaaaabaabaabbb", "bbaaabbbbaaaabbbaaabbaaa", "bbabaaabbaaaaaaabbabbaba", "bbabaabaaabaaabbbaaabababaaaabaa", "bbbbababbbbabaaababbbaaaababababbaabbbaaabaabbaaaaabbbbb", "bbaaaaabbbaaabaabaababab", "aaaabaaabaaabbbaaababbab", "aabbaababbabbbbbabbababa", "baaaaaaaaabbaabaaabbbbabbaaaaaababaababb", "aabbaaabababababaaaaabbb", "aabaaaaabbbbaabaaaaabaab", "bbaaaaabbbbabaaaabbbabba", "babaaaababbabbbbbbbaaaaa", "bbbbaabaaaabbbbababbaabaabbbababaabaaaabbaababba", "bababbbbbabbbaaabbabbaba", "abbaaaabbabbbaaabaabbabb", "aabbbababaaaababbabbbbab", "abaaabaabbbbabababbbaaababbabaaababaabba", "bbbabbabaaabbabbabbabbbabaaababbaaaababababbbbabbabbabaaabaaabaaaaaabaaababbaabb", "abbbaaabbabaaaaabababbbabababbbbabaabbaa", "aabaaaaabaababbbbaaaaaba", "aaaaaaabbabaaaababbbbaab", "aabaaababbaaabbabaaabaaaaabbaaaababaababbbbbbbbbabaaaaab", "bbbbbbbbbbaabababbbbbbbbaabbabbb", "abbbbbbaaabbbbbbaaaaabaabbbbababbabbabab", "baaababaabbbaaabababbbbb", "bababbbabbabaaabbbabababbbbbabbaabbbabbb", "baaabbbabaabbabbbbabbaba", "ababbbbabbaaaabbbaababbbaaabbbbbbbabbbabaabaabaabbaabbaabbbaabbaaabaabba", "bababbbaababbabbaabaabaabbbbaaab", "aaabaabaaabaabbabbaabbaaabbbaaab", "abaaababbbbbbaabbaabbaab", "aaabbabbaaaaaabbaaabaabb", "bbbabbabbbbabaabbbabbbabbabbaabbabbaaabb", "bbaababaabbaabaaaabbbbba", "ababaaaabaabbbaaaaaababb", "babaabababaaabaabbbabbbbbbbbbbbbbabaabbbabbbbbaaabbaababbaaabaababbbbaba", "ababbabbbaababababbababbbbabaabaababbabbaabbbbaa", "baaaabababbaababaaabaaaaaaabbbaabbababbabaaaaaabbaaabbaaaabaaaaababbbbababbabaab", "aaabbbbaabbabbbbbababaaabababbbbabaabaabaabbbaaaabbbbaab", "aabbbbbbabbaaaabaaabaabb", "bbbaabbbaaaaaaabbbaabaabbababbbaabababbaabbaaabb", "bbbbaaaababbbabababaaabb", "bbaaabbbbababbbababbbaab", "bbabbabbaabbbbabaaaabababaababaa", "abaaabaaabaaababbaababaa", "aabaaabbbaabaaaabbbbbbab", "baabaaabbabaabababbbabaa", "ababbabbbaabbbbbbabbabaa", "abbbbaaabbbabbbbbababaaa", "bbbbbbaabababaaaabaababa", "aabbaabaabaaaabbbaabbaba", "bbbbbbaaaabbaaaaaabbaabaaaaaabbb", "aaaabbbbaaaaabaabaaaaaabaaabaabb", "abaaababbaaaababaaaaaaaaabaabbabababbaab", "babababbabbabaabaabaabbb", "babaaaabbbabbabbbaababab", "aaabbababbbbbbbaabbbbabbbbbbaabbaaabbabbaaaabababaaabbaaababbaab", "abaabbbabaaaabbbabbbababbaaaabbbbabbabaa", "aabbbbaababbaababbbaabaa", "bbaabababbaababaaaabbbaa", "babaababbbbbabaaaabaaabaabbabbbbaaaaaabbbbaababbabaabaaaaabbbaaababbbbbb", "baababbbbaaaaaaabbabbaab", "aaaabbbaababababbbbbbabb", "bbaaaaaaababbbaaaabbabbabbabaaababbbbbbabbbaaaaabbaababbbaababaa", "aaaaaaabbbaaabaabbbabaabbbabaababbaaabaabbaababb", "babaaaabaabbbbaabaaaaaabbaaaaaba", "aabbbaabababbbabbabaaabababbbbbabaababbaaabbaabaaabbaaaabaabbbbbbaaaababbbaabaab", "babaaaaaababbbabaabababb", "babbabbbabbaababbabbbaab", "baabbbabbabbbabbabbbbaaaaaaaaaaaaabaabbaaaababbbabbbaabb", "bbbaabbbbababbabbbbaaabb", "babaabbbbaabaaabaaabababbbaabbbbbbbabbba", "bababbabbaaabbbabbbbbabb", "bbabbbabbbabbbbbbbbaaaab", "baabaaaaabbaaaabababaaaaaaabbaaa", "ababbbaabbabbabbbaabbbba", "abbaabbbaaaabbbbaaaaabba", "bbaababbbbababaaabbaababbabbabaababbbbab", "bbbabbbbaaaaaabbbbaabaaababaaabbaaaababb", "baaaaaabbbbbbabbbbaabbaaababbbbb", "abbbbbbbababbaaaababaabababbabbaabaaabaababaaaaaabababab", "ababababbbaaaaaabababbbbabaaabbb", "baaabbabbbabbbbbbbaaaaabaabababa", "baaababaabbaaaaaabababaababbaababaaaabbbbbbbbaaaabaabbaa", "abbbbbbaababbaabbababaaaaabbbbbaaababbbbaaabbbbb", "aaababaaabaaabaaabaaabbb", "baabaaaabbbbbbaabbaabbba", "ababbbabbbbbabbababbabab", "bbbababaababbbaaaaaaaaaaaaaabababaababab", "aababbbbbabababbbbaaaabb", "bbaaaaaabbabaabaababbbba", "bbabaabaabbabaabbaabbabb", "abbbabaabbbbbbabaaaaabaababaabab", "baabbbaabbbababaaaaabbab", "babaabababbaabbbabaabbbb", "aabaaaaaababbabbabaabbbb"]
  in  "Input":string="62: 110 112 | 92 68\n85: 38 92 | 102 110\n63: 92 6 | 110 23\n82: 110 | 92\n99: 110 122 | 92 54\n33: 110 61 | 92 103\n24: 110 92 | 110 110\n76: 3 92\n109: 26 92 | 81 110\n94: 92 78 | 110 28\n17: 110 115\n61: 92 110 | 110 82\n25: 9 110 | 61 92\n114: 47 110 | 63 92\n21: 30 82\n103: 82 82\n69: 5 110 | 43 92\n73: 110 116 | 92 69\n52: 92 81 | 110 103\n22: 119 92 | 50 110\n108: 37 92 | 35 110\n2: 71 92 | 20 110\n119: 103 110 | 88 92\n102: 101 92 | 49 110\n92: \"b\"\n91: 92 54 | 110 3\n64: 92 115 | 110 24\n68: 92 30 | 110 81\n89: 115 110 | 26 92\n80: 61 110 | 81 92\n19: 110 73 | 92 1\n16: 115 92 | 103 110\n15: 123 110 | 58 92\n115: 110 110 | 92 110\n70: 92 30 | 110 9\n40: 110 96 | 92 99\n50: 88 110 | 115 92\n18: 26 92 | 48 110\n81: 92 110\n107: 110 30 | 92 115\n38: 84 110 | 12 92\n44: 40 92 | 66 110\n27: 125 92 | 2 110\n41: 92 128 | 110 118\n56: 81 92 | 30 110\n88: 110 92\n13: 75 92\n55: 75 110 | 26 92\n12: 13 92 | 52 110\n28: 122 92\n121: 75 92 | 24 110\n113: 92 81 | 110 54\n98: 103 110 | 3 92\n6: 92 62 | 110 126\n96: 75 92 | 9 110\n9: 82 92 | 92 110\n0: 8 11\n32: 104 92 | 91 110\n116: 110 32 | 92 67\n104: 92 81 | 110 30\n5: 110 109 | 92 105\n117: 110 22 | 92 59\n128: 92 24 | 110 9\n66: 92 98 | 110 21\n46: 76 92 | 89 110\n36: 92 90 | 110 127\n20: 110 115 | 92 3\n4: 48 110 | 30 92\n26: 92 82 | 110 110\n39: 30 110 | 115 92\n127: 61 110 | 9 92\n84: 110 104 | 92 78\n100: 97 92 | 68 110\n106: 110 7 | 92 18\n123: 110 64 | 92 68\n111: 110 74 | 92 46\n42: 114 110 | 19 92\n58: 28 92 | 16 110\n47: 110 15 | 92 124\n54: 92 92 | 110 92\n51: 110 117 | 92 111\n130: 92 41 | 110 106\n30: 92 92 | 110 110\n72: 17 110 | 109 92\n129: 130 92 | 108 110\n14: 85 110 | 51 92\n53: 87 92 | 44 110\n112: 92 30 | 110 122\n45: 61 82\n105: 75 92 | 61 110\n90: 110 122 | 92 9\n122: 110 92 | 92 110\n83: 110 33 | 92 56\n118: 110 61 | 92 75\n74: 120 92 | 78 110\n29: 110 65 | 92 60\n31: 14 92 | 10 110\n110: \"a\"\n87: 36 110 | 94 92\n57: 92 48 | 110 81\n78: 92 115 | 110 54\n97: 92 48 | 110 122\n1: 110 27 | 92 34\n95: 92 107 | 110 86\n79: 110 55 | 92 77\n37: 92 109 | 110 25\n126: 4 110 | 39 92\n101: 45 92 | 80 110\n59: 110 70 | 92 105\n7: 61 92 | 48 110\n48: 92 92\n35: 104 92 | 57 110\n120: 48 92 | 48 110\n34: 29 110 | 79 92\n93: 54 92 | 26 110\n71: 115 110 | 61 92\n125: 121 110 | 45 92\n60: 122 92 | 54 110\n86: 54 110 | 9 92\n49: 97 110 | 91 92\n3: 110 110\n23: 110 95 | 92 72\n65: 92 103 | 110 115\n10: 129 110 | 53 92\n8: 42\n11: 42 31\n77: 103 92 | 81 110\n67: 93 92 | 112 110\n75: 92 110 | 92 92\n124: 83 110 | 100 92\n43: 92 113 | 110 56\n\nabbabbbbaaabbbbabbbababaaabaabaabbaabbba\nbabaaaabbaaabbbbbbbbbaba\nbbbbaaaabaaabbabaababbbabaaaaaababaabaaaaabbabbb\nbaabbbbbbbaababaababbbabbababbbbaaaabbbbbabaabbabaaababb\naabbaabbbbbaabbbbaaabaab\nbbaaabbaaaabababbbbaabaa\nabbbbbababbaabaabaaaabbbaaaabaab\nabaabbbbabaaabaabbbbaabbabaabaaabbaaabbbabbaabbbaabbbabb\nbaabbbbbaabbaaabbabbabaa\nbabbabbbabaabaaaaabbababaaaabaaaabbababbabababbaaababaaa\naaababaabababbbbabaaaaab\nbbabaabaabbaabaabbbbbbab\nbbbbaaaabaaabbabbbbbbaababaabbaabaabbaab\naaabbabbbabababbaabbabba\nabbbbbbabbababbbbabbabbabbabaabbaaabbaab\nbbbbabaaabbaabbabaaabbbababababbabaabbaabbabbbaa\naabaaaaabaabaaabaaabbaababbbaaababbbbbbabbbbabababbbabbaabaaabaa\nbaaaababbaaaaaabaabbbabbaaabaaab\nabbabbbaaabaaabbaaaaabbb\nababaaaababaaaaaaababbaa\nbabbabbabbababababbaaabb\nbbabbaabaaabbabbababaaababababaaaaababaabbaababb\nbbababbbbbabaaabaaabaaaa\nabbaaabaaaabaabbbbbaaaba\naaaabababbbbabaabaabaaabbabbabbabaaababaaabaabbaabaaabbabbaaaabababbbaab\naabaababaaaaaabbaabaaabbbabbbaaabaabaaaaabbaaaba\nbababaaaabbaabbbaaaabbab\nabababaabbbbbaababbaaaabbabaabbbabbbbaaaabaaabbbabbbbaba\nababababababbbaaababbbba\nababbabbabaabbbaabaaaabbaaaaaaaaaaabaaaabbbababb\naaabbabbbaaabaaaabaabaaa\nabbbbabbabbbbaaabbbbabbbbabaaaababbbabaababbaabbabaaabba\nbbbababaaaaabaaabaabaaabbaababba\naaaabbbbbbabababbbaaabab\naabaababbbbbaabaabaaabaaabababbbbababbabbbbabbaa\nbabbabbaabababaaabbbabaa\nbaaaaaaabbabababbbaabaaa\naaababaaaaabaaaaabaaabbaabaaaaab\nabaaabaabaaabaabaaabaaaabbaabaaabbbbbbab\naaabbbabaababbbbbaabaaba\nbababbbaabababaabababaab\nbababbbaaaabaaaabbbaaabbabbaaabb\nababaaabbababaaabbabbbbabaabaabaabaababb\nbbabbaabbabaabbbabbabbbaaabbaabaaaaaaaababbbbaaaabbaabab\naaababababaaaabbaaaaabba\nbabaababbbbabababaabaaaaababbabaabaaabba\naaaabaaaabababaaaaabbaaa\naabaaaaababbbaaaabbbabababbabbaa\nbbbbaababaabbbabbbbabbaa\nbaaaaaabaabaaaaaabbaabbaabbabbbbbbbabbabbbbbabbbabaabbab\nababababbaaaaaabaabaabbb\nabbbababababbbaababbaabb\naabbaaabaabbaabbaaaaaabbbbaaabbaabbbaaaa\nbbabbbbaaababaababbbbbbaabbbbbabbabbabbb\nbabbbabaabaabbbabaabbaab\nbbabbbabababbbabaababbbaaabaaaababbbbaba\nbabbaaaabbbabbbbabbaaaba\nbbbbababbbababbbbbabbbabbbaabbbbaaabbaaa\nababbbaababbbabaaaaaaabaabaaaaaabbabaabbaaaaaabababaaabaaaaaababbbbabbbbaababbaabbbbaaab\naabbbabbaabbaabbbaaabababaaabaabbbabbaba\nbbbabaabbbabbaabbaabaaaababbababababbbba\nabaabbbabaaaaabbabaaabbb\nbababbabaabaabaaaabbbbaabbababba\naabbaaabaabbbabbaababaaa\nbaababbbbbabaabaaaaabbab\nbbbbabbaabbbbbbbabbbaaaaaaabaabababaaaaaabababbbbaababab\nbaaaabbabbaaaaaababaaaaaabaabbbbababbbbb\nbaababbbabbbbaaabbaabaaa\nbbbabbabbbbbabbbbaaaaaaaaaabbabaabaababb\nbbbbbbaabaabbbaaabbbaaba\nbbbababaaabbbbbbbbbbababaabaabaababbbbba\nabbaabbaabbaaaababaaaaababaabaaaaabbbaabaabaaaabaabbabbbbabaabba\nbaaaabbbaaabbaabaabbbabababbaaab\nabaaabaaabababaababbbbbb\nbbbbaaaabbabaabaabaaabaabaabbaaa\nbbaaabbbbaaaaaaabaabbbbbbbbaabbbaaaaabbb\nabbaabbabaaabbabaaabbbbabbababba\nbaabaaaaaabbabaaaabaabbbbaabbaab\nbabbbababaaababaabaabbaa\naabbbbaaababbbaaabaaaaab\nbbaaabbbaabaaabaabbbabba\nbabbbaaabababaaababbbaab\naaaaaaaaabbbababaaabbaab\nbbaabaabbabbbaaababbbaaabbbbbaabbbababba\nababababbaaabbabbababbbbbbbbabba\nabbaabbababbbabaabbabbbabbaaaaababbbabababaabbaa\naabbbabaaaabbbbbababbbbbbabbaaabbabaababaabbabab\nbabbbaaababaabbbbbbabbaa\nababaabaaabbaaababaabbbb\naabaabaaaabbbbaaaabbabaa\nbaaaabbbbbbababbaabaababaabbabaaababbbbabaaabbbbbbbaaabbabbbbbbaaaaaaabaaaaaabbbbbbaaaba\nbaaabbabbabbbabaaaabaaba\nbaaaabbbbbbbbaababbbbbbb\nbaaaabbaaabbbbbbaababaaa\naabaababbaaaababaabbabba\naabbbbaaaabbaaaabaababba\nbbaaabaaaaaabbbabbabaabababbabbaaababbababaabbab\nabbabbbaaabaaabbabbabbaa\naaaaabbbbbbbbbbbabaababbababbbbabbbabbbaabaababb\nbbbbababbbabaabababbbabaaabaabababaaaabbabaabbabbbaabbab\nbabbbabbbababbbbabbaabbbabaaaabbbbabbaabaabbabaaabbbbaab\nbaabaabbaaababbaaababbbbbbaaabbbabaaaaabbbbbaaabbbbaaaaa\nabaaababaaaabababbaabbab\nabababaaaaaabaaababbabba\nabbbaaabbaabbbbbbaaababb\nbaabbbbbbbbbabbbbbaabbba\nabaaabaaabbbbbabbbbabbba\nbabbbabbaabaabaaabaaaaaa\naaabbabbabaaababbbbabbabbabaaaabaabbababbbbbabba\naabaaaaaababaaaabababaaaabbbbbbababbaabaabbbaaaa\nabaaaabbbbbabaaaaabbbbababaabaaa\naaabbbabaaaabaaaabbabbab\nbbbbaabbbabbbabbbaaabbbabaabaabbbabbabbbabaaabbaabbababb\nbabaabbbbbbbababbbaabaababbaaabb\nabbbbabbbbbbbbbababbaabb\nabaaaabbaabbbbaabaabbbbbbabbabbababbbbbbabbabbaabababaab\naaabbabbaaaabbbaabbbabaa\nbabbbabaabababaaababbaba\nabbaabbababaaaaaaababaaa\naabbbabbabababbbabbbbbaa\naababbbbbaaaaabbbaabbaab\naabbaabaaabaabaaaabbbaab\nabaabbbabababaaaaabababb\nabbbbbbaabaaabaababbabbb\nbaabaaaaaaabbabaaabbaabbaabbaaab\nbaababbaababbaabbbbabbaa\nababababbabaaaabbaaabaab\nabbabbbbabbbababaabababb\nbbabbabbbbabaaabaabbbbba\naaaaaabbbaaaaabbabbababb\nbaaabaaababbbabaaababbbbbbaabbab\nbbbbbbbababaababaababbaa\nbaaaaaaaabaabbbaababbabbbaaaaaabbaabaaaaababbbbaaabaabaa\naaabbbabbaaaabbbbabbbabababaaabababaabba\nbbbabbabababbabbbabaaabb\nbbaaabaaaaaaaaaababaaabb\naabaabbaaabbbaabbaaabaaaababbaab\nabbbbaaabbabbbbbbbbbbbaabbabbabbbabbbbab\naaababaabaababaabbbaabab\nbaabaabbbbabbbabababbaaa\nabbbaaabaabaababbbbbababababbaabbabaaaaaabbbbbaa\naabbbbbbbbbabbbbabaabaab\nbababaaabbbabbbbababbaba\nbbabaabbbababaaabaaaaabb\nbbbbbbaababaababababbbbb\nbababbbbabbbbbabbaabaaba\naabaababbbbbbbbabaabbbabbbabbbabbbabbaabaabaaabbababbaba\nababbbabbaaabbabababbbbbababaabaaabaabaabbbaaaaaaaaabbaabbbababbaaabbabbbbaabbaa\nbbabbbabaaabbabaabaabaaa\nbbabbaabbbaaaaabababbbbb\nbbbbbbaaababbabbaababbaa\nbbbbbbaabbabababaaaabaab\nabbaaabbabbababbabababbaaabbbbababbaabbbabbbbbab\nbbbbababbabbbabbbbaabaaa\nbbaabaabbababbaaaabbaaaabaaaaaba\nabbaabaaababbabbabbbabaaaaaabaab\nbaaaababbbabbabbbbbbaabbabbaaaaabaabbbaaaaabbaaaabaaaaab\nbbbbbbbabaabaaabbbabbbbaaabbbbababbaaabb\nbbaaabaaabbaaaaaaaabbaaa\nbabaabbbabbabbbbbaaabbbbababaabb\nbbbbabbbbababbbabbabbbaa\nbaaaaaababbaaaabbbbaabba\nabbbaaabbbbbababaabbbbbb\naabbaaaaaababaabbabaabbbbabbaabaaaaaaaaaaababbab\naaabbabbbbbabababbbbbbab\nbabaabaabbbabaaaaaabbababaababba\nabaabbbaabbbbbababaaaaab\naaabbabbaabababbaabbbbba\naabaaabaaaaabbbaabbbaabaababbbbbbbbbaabbbbbbaabbbaabbaaa\nabbaabbbbaaaabbbabbbaabb\nbbaaabbaaaababaabbbabaababaaaabaaabbbaabbbaababbbaababba\nbabaababbabaaaaaaaaaabaabbbbbaababbabbaa\nbbaaabbabbabbbabaaaaabbb\naaaabababbababbbaabbbbababbaaaaabaaaaaba\nbbabaabbbbbbbbbaabaaaaab\nbbabaaababaaababbaaaabaa\naabbaaabaabbbabaabbbabaa\nbababaaabbbbbbbabababaaaabaaaaab\nabaaaabbaaaaababaaaaaaba\nbaaaabbaaaababababaabaabbaaaaabbbaababba\nbbababbbbbaaaaabaabababb\nbbbabbbbbbbbaababbbbaabaabbbbbaa\nbbbabbbbabaabaaaababbbbaababaabb\nbbbbababbabbbabbbabbabaa\nbaaabababaabbbaabbabaabababbabbaabbaabab\naaababbabaaaaaaabbbaaaba\nbaaaaaabaabaaabaaabaabba\nbabbaabababababbaaabbaaa\nbbbababaaaaaaaabbbbaaaab\nbababbaabbbabaabbaaaaaba\nabababbbbbbbabababbabbaa\naaabbbabbaaabbabaabababa\naaaabbbababaabbbabbaaaaaabaababbbabbabab\nbbaaaaababaaabaababaaaabbabaabbbaaaabbaa\nabbabaabaabbaaabbababbbabaaabaab\nabbbababaaabbabbaaabbaab\nabbabbbbabaaababaaabbbaa\naababaababbaabbbaababbaa\nbabaabaaaaabaaabbbbbaaab\naababbbbbaababbbbaabbabb\nbbbbaaaaabaaaaabbbbaabaabbababbabaaabbaabbbaabab\nababababbaaaabbbbbbaabbbabbbbbaa\nbbabbbbbbbababbbbabbabab\nbbbbbbbbbbabbaabbabbbaaaaabbbabaaabbbbba\nbbabbbabaabbaaabbbbabbba\naabaabbbbbaababbaabababa\nbbaabaabbbbbababbbbbbaaa\nbababbaaaaaaaabbabbbbaaabbbabaababbbbababbabbbaaabbbaabb\naabbbbbbbbbbabaabbbbbaaa\nababbbaabbbaabbbbaaaaaabababaaababbbababbbabababbbaabbbb\naabbbbbbbaabbbabbbabbaaa\nbababbababaaaabbabaabbab\naababbbbababababaaabbaaa\nbbbbababbbabbbabbaababaa\nabbbbaaabbaaabbbbaaaaabbaaaaabba\nabbaabbabbaabaabbabbaabb\nbaaaabbbaaabbbbabaaabaab\nbaaabaaabbaababaaaabbaab\nbaabbbabbbbbbaabbabaabbbbaababab\nbbabababaaabbbababaababa\naabaabaabbabbbbababbaaababbbabbbaabbabaabbbbabbabbbbbbbb\nabaaaababbbbababaabababb\nabbabbbbaaaabbbbabbabbbbababaabb\naababaabaaaaabaababaaaba\nabbbbaaabbaaaaabaaabbaaa\naabaaabaaabbaaaaaaaabaab\nbbaaabbbbbbababaaabababa\nbbbabbabbaaaababbabaabbbaabbbbbbabbaaaaabbababba\nbbbbababbaaaaabbabbbbbabbaabbabb\nbbabaabbbbbbaabbbaabbbabaabaaaaabaabbaaa\nabbaaaabbbbbabbbabaabaaa\naaabbbbaaaababbabaaaaaba\nbababbaabaaaabbaaaabbaaa\nababababaaaabaaaababbaab\naabaaababbabaabaabaabbbb\nabbaabbbbbbbabbbbbbbbaabbbababbbaaabbaaabbababaa\nabbabbbbaaaabaaababbbabaabbbabaaaabbabaa\naababbbbbaabaabbbbbabaabaababbbbbbbbaaabbbabbaaa\nbabaaaabbbabbaabbaababba\nbbabbbabbbbbabaabaaaabaa\naaaaaabbaabbbababaaabaab\nabaaaababbbbbbaaabaabaab\nabaabbbabaaaaabaaaaabbaaaaaababbabbbaabb\nbbbbaaaaabbaabbabbbbabbbbbabaabaaaabaaab\nbbabaaabaababbbabbababbbababbaaa\nbbbbbbbbbbabaaabbaabbabb\nbbbabbbbabbaabbbbaababbbabbababb\nbbaaabbabaabbbaabaababab\nbbabaabaabbbababbaaabbabbbbbaaab\nabbbbaaaababababbabaabbbabbbbbbb\nbabaaaaaaabaaabababaababbabbaabbbbaabaaa\nbaaaabbabbaababaabbababb\naaaaaaabbaaaabbbbbbaaaaa\naabaaaaabbbabaabbaababaa\nabbabaabbbabbbbbbaabaaaaaaaabbaaaaabbaab\nbaaaabababbbbaaabaababaa\nbabaaaaabaaabbbbaaabaaaa\naaabbababaaaaaaaabbbabaa\nbbabaaabbaaaababaaabaaaa\nbbaaabbbbabbbbbaaabbbbbaaabbbbbabbabaabababbbbbaabbabbaabbbabbbaaaaaaaababbbbababaabaabb\naabaaaaaaabababababbabaaaaabbaaa\nbbbabaaabbaaaaaabbbaaaab\nabaaaaaabbabaaaabbbaabbabbababaa\nbbaaabbaaabbbabaababbbbb\nbbabaaabbababbbababaaaabbabaaaba\nabbabbbabaaabbbaaabaaaab\nbaaabbbbbabbbaaabbbaaabb\nbbaaabbaababbbababaaabba\naaaaabaaaabbbbabaabbbbaaaababbbbbabaabbbbbabbbaa\nbbaaaaaaabababbbbabbbbaa\nababbabbaabaaaaaaaababbb\nbabbabbabaabaaabbabaababbbbaabbbbbababababaababb\nabbaaaaabababbbbaaaabababbaaaaabaabaabbb\nbbaaabbbbaaaabbbaaabbaaa\nbbabaaabbaaaaaaabbabbaba\nbbabaabaaabaaabbbaaabababaaaabaa\nbbbbababbbbabaaababbbaaaababababbaabbbaaabaabbaaaaabbbbb\nbbaaaaabbbaaabaabaababab\naaaabaaabaaabbbaaababbab\naabbaababbabbbbbabbababa\nbaaaaaaaaabbaabaaabbbbabbaaaaaababaababb\naabbaaabababababaaaaabbb\naabaaaaabbbbaabaaaaabaab\nbbaaaaabbbbabaaaabbbabba\nbabaaaababbabbbbbbbaaaaa\nbbbbaabaaaabbbbababbaabaabbbababaabaaaabbaababba\nbababbbbbabbbaaabbabbaba\nabbaaaabbabbbaaabaabbabb\naabbbababaaaababbabbbbab\nabaaabaabbbbabababbbaaababbabaaababaabba\nbbbabbabaaabbabbabbabbbabaaababbaaaababababbbbabbabbabaaabaaabaaaaaabaaababbaabb\nabbbaaabbabaaaaabababbbabababbbbabaabbaa\naabaaaaabaababbbbaaaaaba\naaaaaaabbabaaaababbbbaab\naabaaababbaaabbabaaabaaaaabbaaaababaababbbbbbbbbabaaaaab\nbbbbbbbbbbaabababbbbbbbbaabbabbb\nabbbbbbaaabbbbbbaaaaabaabbbbababbabbabab\nbaaababaabbbaaabababbbbb\nbababbbabbabaaabbbabababbbbbabbaabbbabbb\nbaaabbbabaabbabbbbabbaba\nababbbbabbaaaabbbaababbbaaabbbbbbbabbbabaabaabaabbaabbaabbbaabbaaabaabba\nbababbbaababbabbaabaabaabbbbaaab\naaabaabaaabaabbabbaabbaaabbbaaab\nabaaababbbbbbaabbaabbaab\naaabbabbaaaaaabbaaabaabb\nbbbabbabbbbabaabbbabbbabbabbaabbabbaaabb\nbbaababaabbaabaaaabbbbba\nababaaaabaabbbaaaaaababb\nbabaabababaaabaabbbabbbbbbbbbbbbbabaabbbabbbbbaaabbaababbaaabaababbbbaba\nababbabbbaababababbababbbbabaabaababbabbaabbbbaa\nbaaaabababbaababaaabaaaaaaabbbaabbababbabaaaaaabbaaabbaaaabaaaaababbbbababbabaab\naaabbbbaabbabbbbbababaaabababbbbabaabaabaabbbaaaabbbbaab\naabbbbbbabbaaaabaaabaabb\nbbbaabbbaaaaaaabbbaabaabbababbbaabababbaabbaaabb\nbbbbaaaababbbabababaaabb\nbbaaabbbbababbbababbbaab\nbbabbabbaabbbbabaaaabababaababaa\nabaaabaaabaaababbaababaa\naabaaabbbaabaaaabbbbbbab\nbaabaaabbabaabababbbabaa\nababbabbbaabbbbbbabbabaa\nabbbbaaabbbabbbbbababaaa\nbbbbbbaabababaaaabaababa\naabbaabaabaaaabbbaabbaba\nbbbbbbaaaabbaaaaaabbaabaaaaaabbb\naaaabbbbaaaaabaabaaaaaabaaabaabb\nabaaababbaaaababaaaaaaaaabaabbabababbaab\nbabababbabbabaabaabaabbb\nbabaaaabbbabbabbbaababab\naaabbababbbbbbbaabbbbabbbbbbaabbaaabbabbaaaabababaaabbaaababbaab\nabaabbbabaaaabbbabbbababbaaaabbbbabbabaa\naabbbbaababbaababbbaabaa\nbbaabababbaababaaaabbbaa\nbabaababbbbbabaaaabaaabaabbabbbbaaaaaabbbbaababbabaabaaaaabbbaaababbbbbb\nbaababbbbaaaaaaabbabbaab\naaaabbbaababababbbbbbabb\nbbaaaaaaababbbaaaabbabbabbabaaababbbbbbabbbaaaaabbaababbbaababaa\naaaaaaabbbaaabaabbbabaabbbabaababbaaabaabbaababb\nbabaaaabaabbbbaabaaaaaabbaaaaaba\naabbbaabababbbabbabaaabababbbbbabaababbaaabbaabaaabbaaaabaabbbbbbaaaababbbaabaab\nbabaaaaaababbbabaabababb\nbabbabbbabbaababbabbbaab\nbaabbbabbabbbabbabbbbaaaaaaaaaaaaabaabbaaaababbbabbbaabb\nbbbaabbbbababbabbbbaaabb\nbabaabbbbaabaaabaaabababbbaabbbbbbbabbba\nbababbabbaaabbbabbbbbabb\nbbabbbabbbabbbbbbbbaaaab\nbaabaaaaabbaaaabababaaaaaaabbaaa\nababbbaabbabbabbbaabbbba\nabbaabbbaaaabbbbaaaaabba\nbbaababbbbababaaabbaababbabbabaababbbbab\nbbbabbbbaaaaaabbbbaabaaababaaabbaaaababb\nbaaaaaabbbbbbabbbbaabbaaababbbbb\nabbbbbbbababbaaaababaabababbabbaabaaabaababaaaaaabababab\nababababbbaaaaaabababbbbabaaabbb\nbaaabbabbbabbbbbbbaaaaabaabababa\nbaaababaabbaaaaaabababaababbaababaaaabbbbbbbbaaaabaabbaa\nabbbbbbaababbaabbababaaaaabbbbbaaababbbbaaabbbbb\naaababaaabaaabaaabaaabbb\nbaabaaaabbbbbbaabbaabbba\nababbbabbbbbabbababbabab\nbbbababaababbbaaaaaaaaaaaaaabababaababab\naababbbbbabababbbbaaaabb\nbbaaaaaabbabaabaababbbba\nbbabaabaabbabaabbaabbabb\nabbbabaabbbbbbabaaaaabaababaabab\nbaabbbaabbbababaaaaabbab\nbabaabababbaabbbabaabbbb\naabaaaaaababbabbabaabbbb"
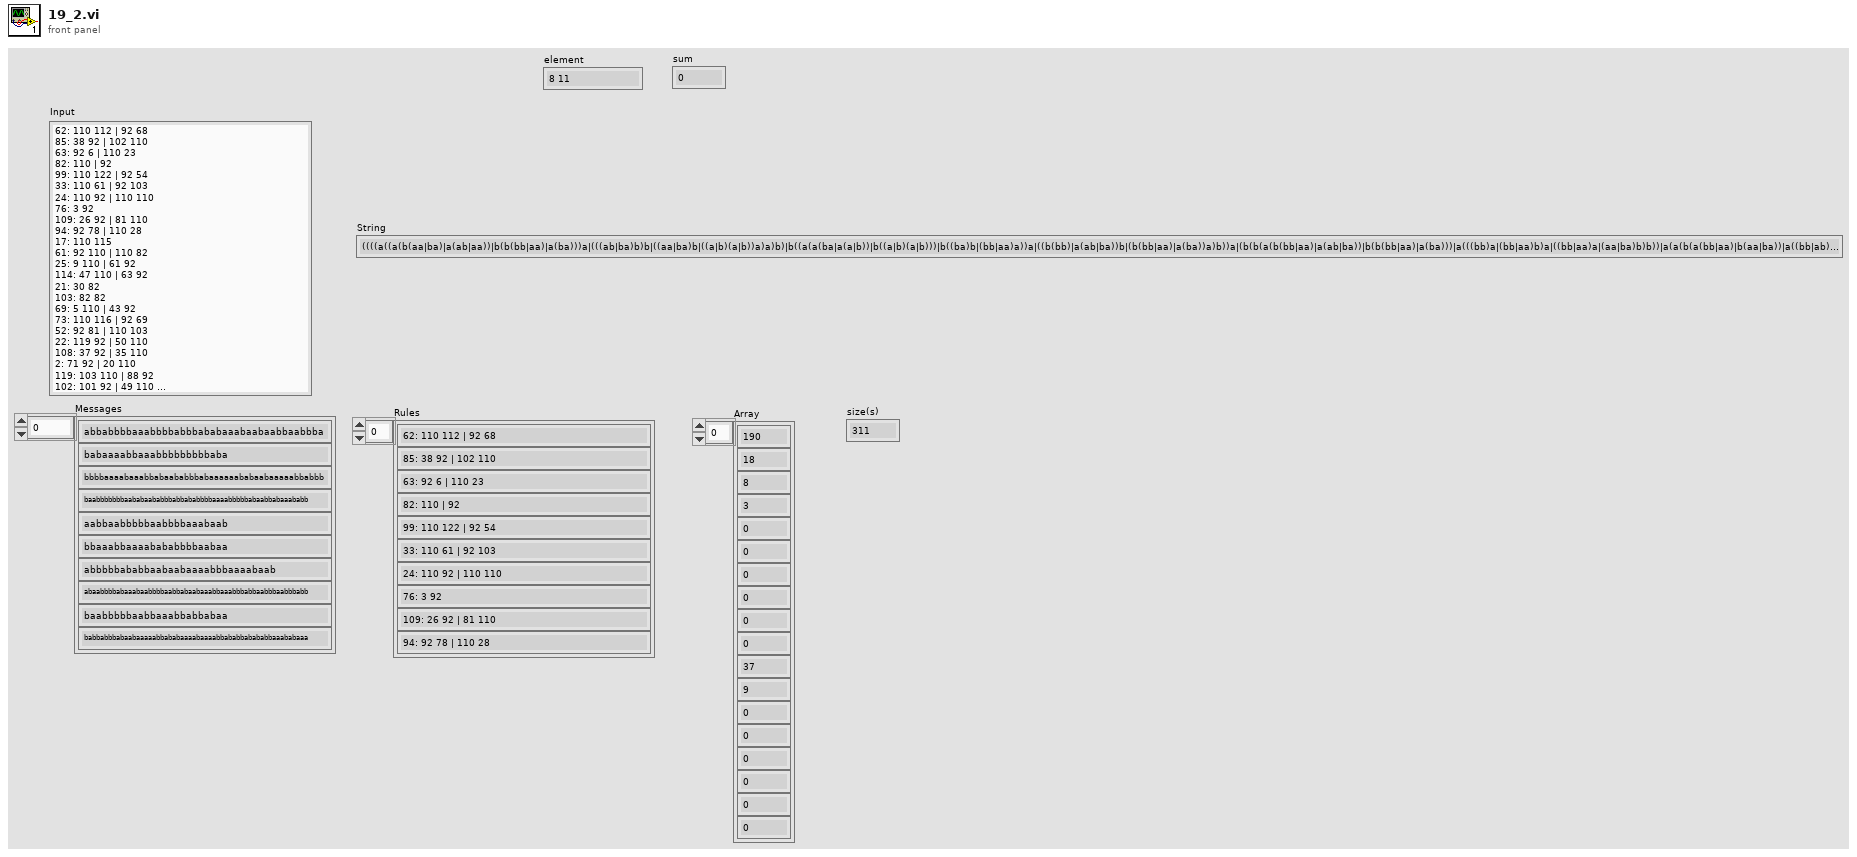
[diagram p1: front panel]
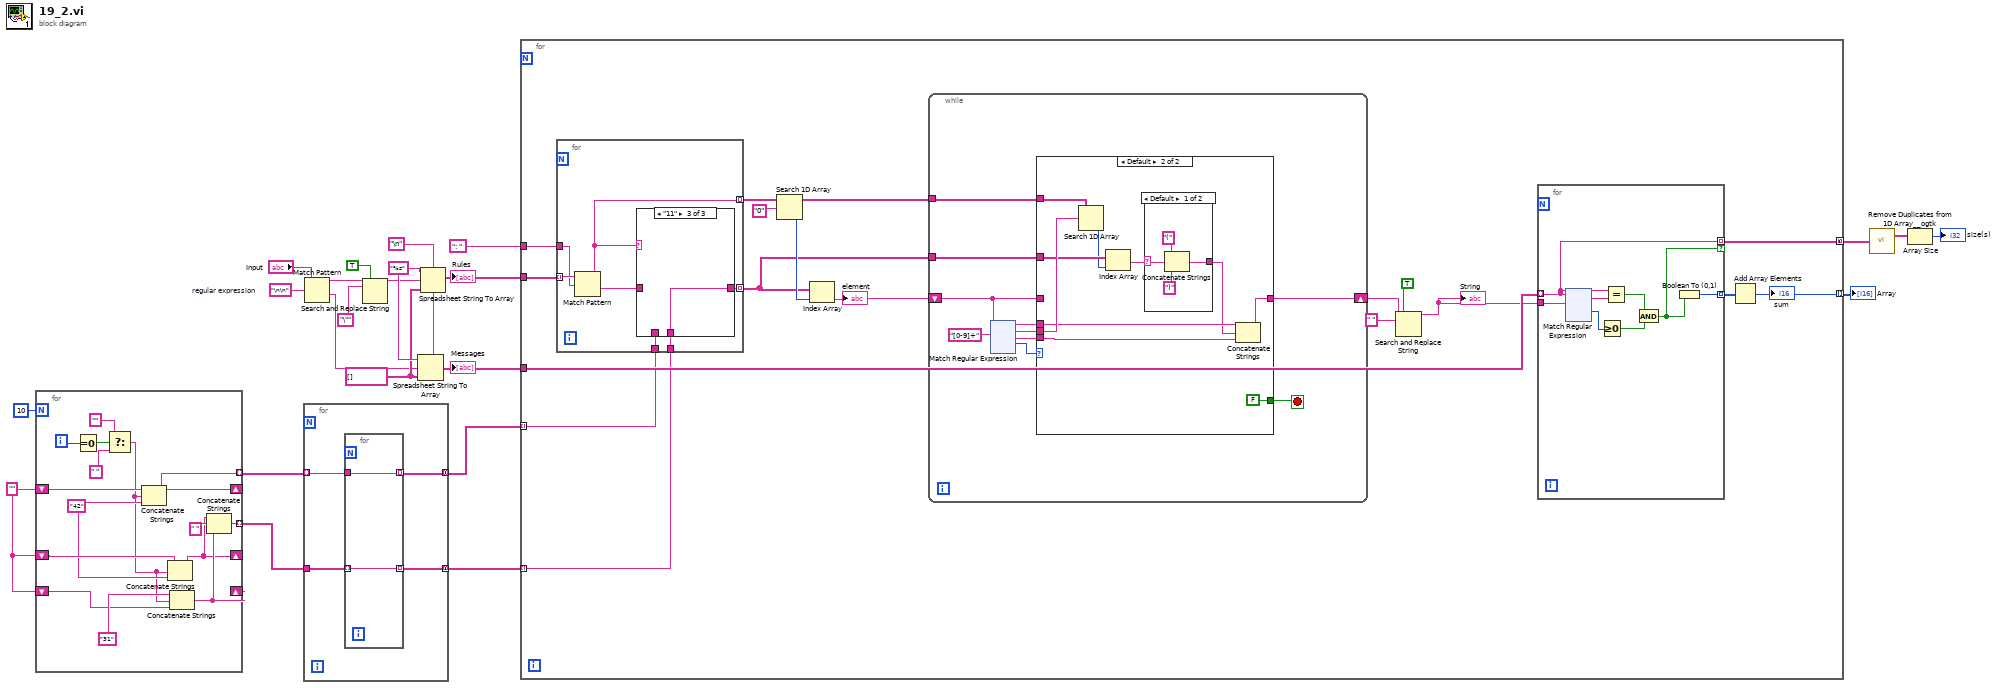
[diagram p0: block diagram]
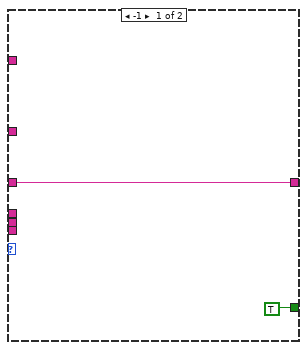
[diagram p4: hidden frame]
diagram:
  w5 = ""
  w19 = "\n"
  w21 = "%s"
  w20 = string[] []
  w22 = "\n\n"  # regular expression
  n1 = for {
    N: 10 -> [_]
    shift-right: [w37] -> _
    shift-left: w5 -> [w38]
    tunnel: [w37] -> w4 mode=indexing
    shift-right: [w25] -> _
    shift-left: w5 -> [w31]
    shift-right: [w26] -> _
    shift-left: w5 -> [w30]
    tunnel: [w24] -> w3 mode=indexing
    i -> [w36]
    w29 = "42"
    n2 = Equal To 0?(x=w36) -> (x = 0?=w35:bool)
    n3 = Select(t="", s=w35, f=" ") -> (s? t:f=w28:string)
    n4 = Concatenate Strings(w38, w28, w29) -> (w37:string)
    n5 = Concatenate Strings(w31, w28, w29) -> (w25:string)
    n6 = Concatenate Strings("31", w28, w30) -> (w26:string)
    n7 = Concatenate Strings(w25, " ", w26) -> (w24:string)
  }
  n8 = for {
    tunnel: w4 -> [w41] mode=indexing
    tunnel: w3 -> [w42]
    tunnel: [w40] -> w2 mode=concatenating
    tunnel: [w39] -> w1 mode=concatenating
    n9 = for {
      tunnel: w42 -> [w43] mode=indexing
      tunnel: w41 -> [w44]
      tunnel: [w44] -> w40 mode=indexing
      tunnel: [w43] -> w39 mode=indexing
    }
  }
  n10 = Match Pattern(string="Input", regular expression=w22) -> (before substring=w15:string, after substring=w16:string)  [unwired: 1 in, 2 out]
  n11 = Search and Replace String(replace all?=TRUE ("replace all? (F)"), input string=w15, search string="\"") -> (result string=w14:string)  [unwired: 5 in, 3 out]
  n12 = Spreadsheet String To Array(delimiter (Tab)=w19, format string=w21, spreadsheet string=w16, array type (2D Dbl)=w20) -> (array=w11:string[])
  "Messages" <- w11
  n13 = Spreadsheet String To Array(delimiter (Tab)=w19, format string=w21, spreadsheet string=w14, array type (2D Dbl)=w20) -> (array=w18:string[])
  "Rules" <- w18
  n14 = for {
    tunnel: w18 -> [w61]
    tunnel: ": " -> [w60]
    tunnel: w11 -> [w54]
    tunnel: w1 -> [w48] mode=indexing
    tunnel: w2 -> [w47] mode=indexing
    tunnel: [w46] -> w10 mode=indexing
    tunnel: [w45] -> w9 mode=concatenating
    n15 = for {
      tunnel: w61 -> [w68] mode=indexing
      tunnel: w60 -> [w67]
      tunnel: [w66] -> w56 mode=indexing
      tunnel: [w64] -> w55 mode=indexing
      tunnel: w48 -> [w63]
      tunnel: w47 -> [w62]
      n16 = Match Pattern(string=w68, regular expression=w67) -> (before substring=w66:string, after substring=w65:string)  [unwired: 1 in, 2 out]
      n17 = case shown="\"11\"" w66 {
        tunnel: w65 -> [w69 _ _]
        tunnel: [w69 w70 w71] -> w64
        tunnel: w63 -> [_ _ w71]
        tunnel: w62 -> [_ w70 _]
        frame Default {
        }
        frame "8" {
        }
        frame "11" {
        }
      }
    }
    n18 = Search 1D Array(1D array=w56, element="0") -> (index of element=w58:i32)  [unwired: 1 in]
    n19 = Index Array(array=w55, index=w58) -> (element=w57:string)
    "element" <- w57
    n20 = while {
      shift-right: [w194] -> w52
      shift-left: w57 -> [w196]
      tunnel: w56 -> [w202]
      tunnel: w55 -> [w200]
      stop <- w195 stop-if-true
      n21 = xnode "Match Regular Expression"("input string"=w196, "regular expression"="[0-9]+") -> ("before match"=w199:string, "whole match"=w201:string, "after match"=w198:string, "offset past match"=w197:i32)  [unwired: 4 in, 1 out]
      n22 = case shown="Default" w197 {
        tunnel: w202 -> [_ w215]
        tunnel: w201 -> [_ w214]
        tunnel: w200 -> [_ w213]
        tunnel: w199 -> [_ w211]
        tunnel: w198 -> [_ w210]
        tunnel: [w205 w209] -> w194
        tunnel: w196 -> [w205 _]
        tunnel: [TRUE FALSE] -> w195
        frame -1 {
        }
        frame Default {
          n23 = Search 1D Array(1D array=w215, element=w214) -> (index of element=w212:i32)  [unwired: 1 in]
          n24 = Index Array(array=w213, index=w212) -> (element=w207:string)
          n25 = case shown="Default" w207 {
            selector: w207 -> [w219 w220]
            tunnel: [w218 w220] -> w206
            frame Default {
              n26 = Concatenate Strings("(", w219, ")") -> (w218:string)
            }
            frame "a", "b" {
            }
          }
          n27 = Concatenate Strings(w211, w206, w210) -> (w209:string)
        }
      }
    }
    n28 = Search and Replace String(replace all?=TRUE, input string=w52, search string=" ") -> (result string=w51:string)  [unwired: 5 in, 3 out]
    "String" <- w51
    n29 = for {
      tunnel: w51 -> [w79]
      tunnel: w54 -> [w73] mode=indexing
      tunnel: [w77] -> w53 mode=indexing
      tunnel: [w73] -> w45 mode=indexing if=w72
      n30 = xnode "Match Regular Expression"("input string"=w73, "regular expression"=w79) -> ("whole match"=w78:string, "offset past match"=w76:i32)  [unwired: 4 in, 3 out]
      n31 = Greater Or Equal To 0?(x=w76) -> (x >= 0?=w75:bool)
      n32 = Equal?(x=w73, y=w78) -> (x = y?=w74:bool)
      n33 = And(x=w74, y=w75) -> (x .and. y?=w72:bool)
      n34 = Boolean To (0,1)(Boolean=w72) -> (0, 1=w77:i16)
    }
    n35 = Add Array Elements(numeric array=w53) -> (sum=w46:i16)
    "sum" <- w46
  }
  "Array" <- w10
  n36 = call-poly <userlib>:"Remove Duplicates from 1D Array__ogtk.vi"("Input Array"=w9) -> ("Output Array"=w8:string[])  [unwired: 1 out]
  n37 = Array Size(array=w8) -> (size(s)=→"size(s)":i32)
